vi "主界面.vi"() -> ()   [LabVIEW 2010]
uses:
  全局量/试验配置信息.vi
  全局量/全局_配置.vi
  全局量/自动测试结果.vi
panel:
  in  "进度提示":string
  in  "加载配置文件列表":u16(ring)
  out "配置文件路径":path
  out "配置文件目录":path
  in  "通道及参数配置":bool
  in  "?":enum32{"板卡类型1", "板卡类型2"}(tab)
  in  "单选_数字量输入":bool
  in  "单选_数字量输出":bool
  in  "单选_DSP输入":bool
  in  "单选_CAN检测":bool
  in  "单选_LAN检测":bool
  in  "单选_R232检测":bool
  in  "btn_数字输出":bool
  in  "btn_DSP输入":bool
  in  "btn_CAN总线":bool
  in  "btn_LAN总线":bool
  in  "btn_R232_485总线":bool
  in  "btn_开始检测":bool
  in  "btn_数字输入":bool
  in  "单选_R485检测":bool
  in  "单选_AD输入":bool
  out "数字量输入检测":bool
  out "数字量输出检测":bool
  out "模拟量DSP输入检测":bool
  out "模拟量AD输入检测":bool
  out "CAN总线检测":bool
  out "LAN总线检测":bool
  out "RS232总线检测":bool
  out "RS485总线检测":bool
  in  "btn_自动开始检测类型2":bool
  in  "函数类型 4":bool caption="y =f4(A1sin(2*π*A2)x+A3)"
  in  "函数类型 3":bool caption="y =f3(x)"
  in  "函数类型 2":bool caption="y =f2(x,A1,A2,t)"
  in  "函数类型 1":bool caption="y =f1(A1*x+A2)"
  out "函数类型4检测":bool
  out "函数类型3检测":bool
  out "函数类型2检测":bool
  out "函数类型1检测":bool
  in  "单选_函数类型4":bool
  in  "单选_函数类型3":bool
  in  "单选_函数类型2":bool
  in  "单选_函数类型1":bool
  in  "进度每次增加数":dbl
  in  "btn_二维码识别":bool
  out "退出？":bool
  in  "btn_退出":bool
  in  "btn_报告管理":bool
  in  "str_测试地点":string
  in  "str_测试人员":string
  in  "str_测试编号":string
  in  "str_报告编号":string
  # "板卡综合测试装置"
  # "板 卡 测 试 信 息"
  # "试验报告编号："
  # "测试板卡编号："
  # "板卡类型："
  # "测试人员："
  # "测试地点："
  # "自动测试"
  # "分步测试"
  # "测试\n项\n目"
  # "分步测试"
  # "自动测试"
  # "测试\n项\n目"
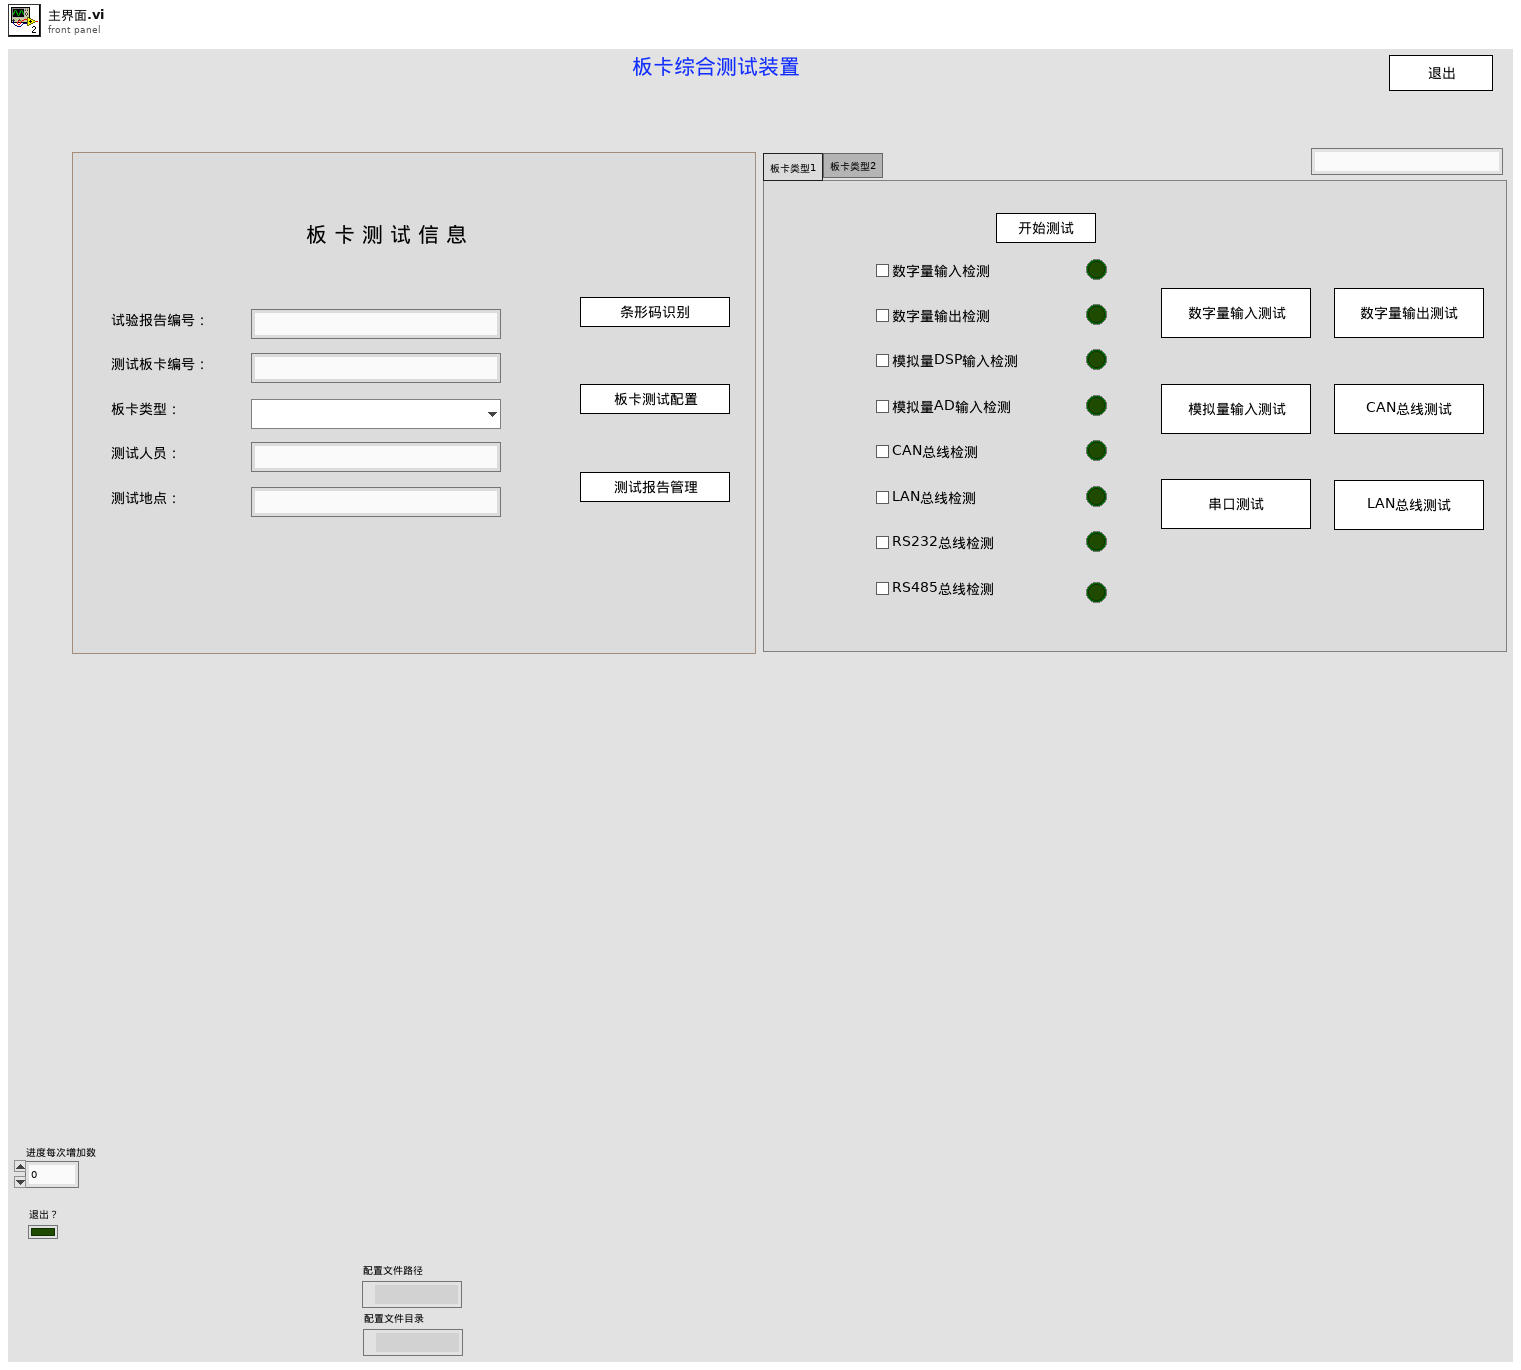
[diagram p1: front panel]
types:
  T1 = cluster{"数字量输入信号路数":i32, "数字量输出信号路数":i32, "DSP模拟量输入信号路数":u32, "DSP模拟量输入信号幅值":u32, "AD模拟量输入信号路数":u32, "AD模拟量输入信号幅值":u32, "RS232端口":u32, "RS232通信路数":u32, "RS232波特率":dbl, "RS485端口":u32, "RS485通信路数":u32, "RS485波特率":u32, "CAN通信路数":i32, "CAN波特率":u32, "以太网选择?":bool, "控制板IP":string, "以太网端口":u32}
  T2 = cluster{"str_报告编号":string, "str_测试编号":string, "RingText.Text":string, "str_测试人员":string, "str_测试地点":string}
  T3 = enum8{"Enabled", "Disabled", "Disabled and Grayed Out"}
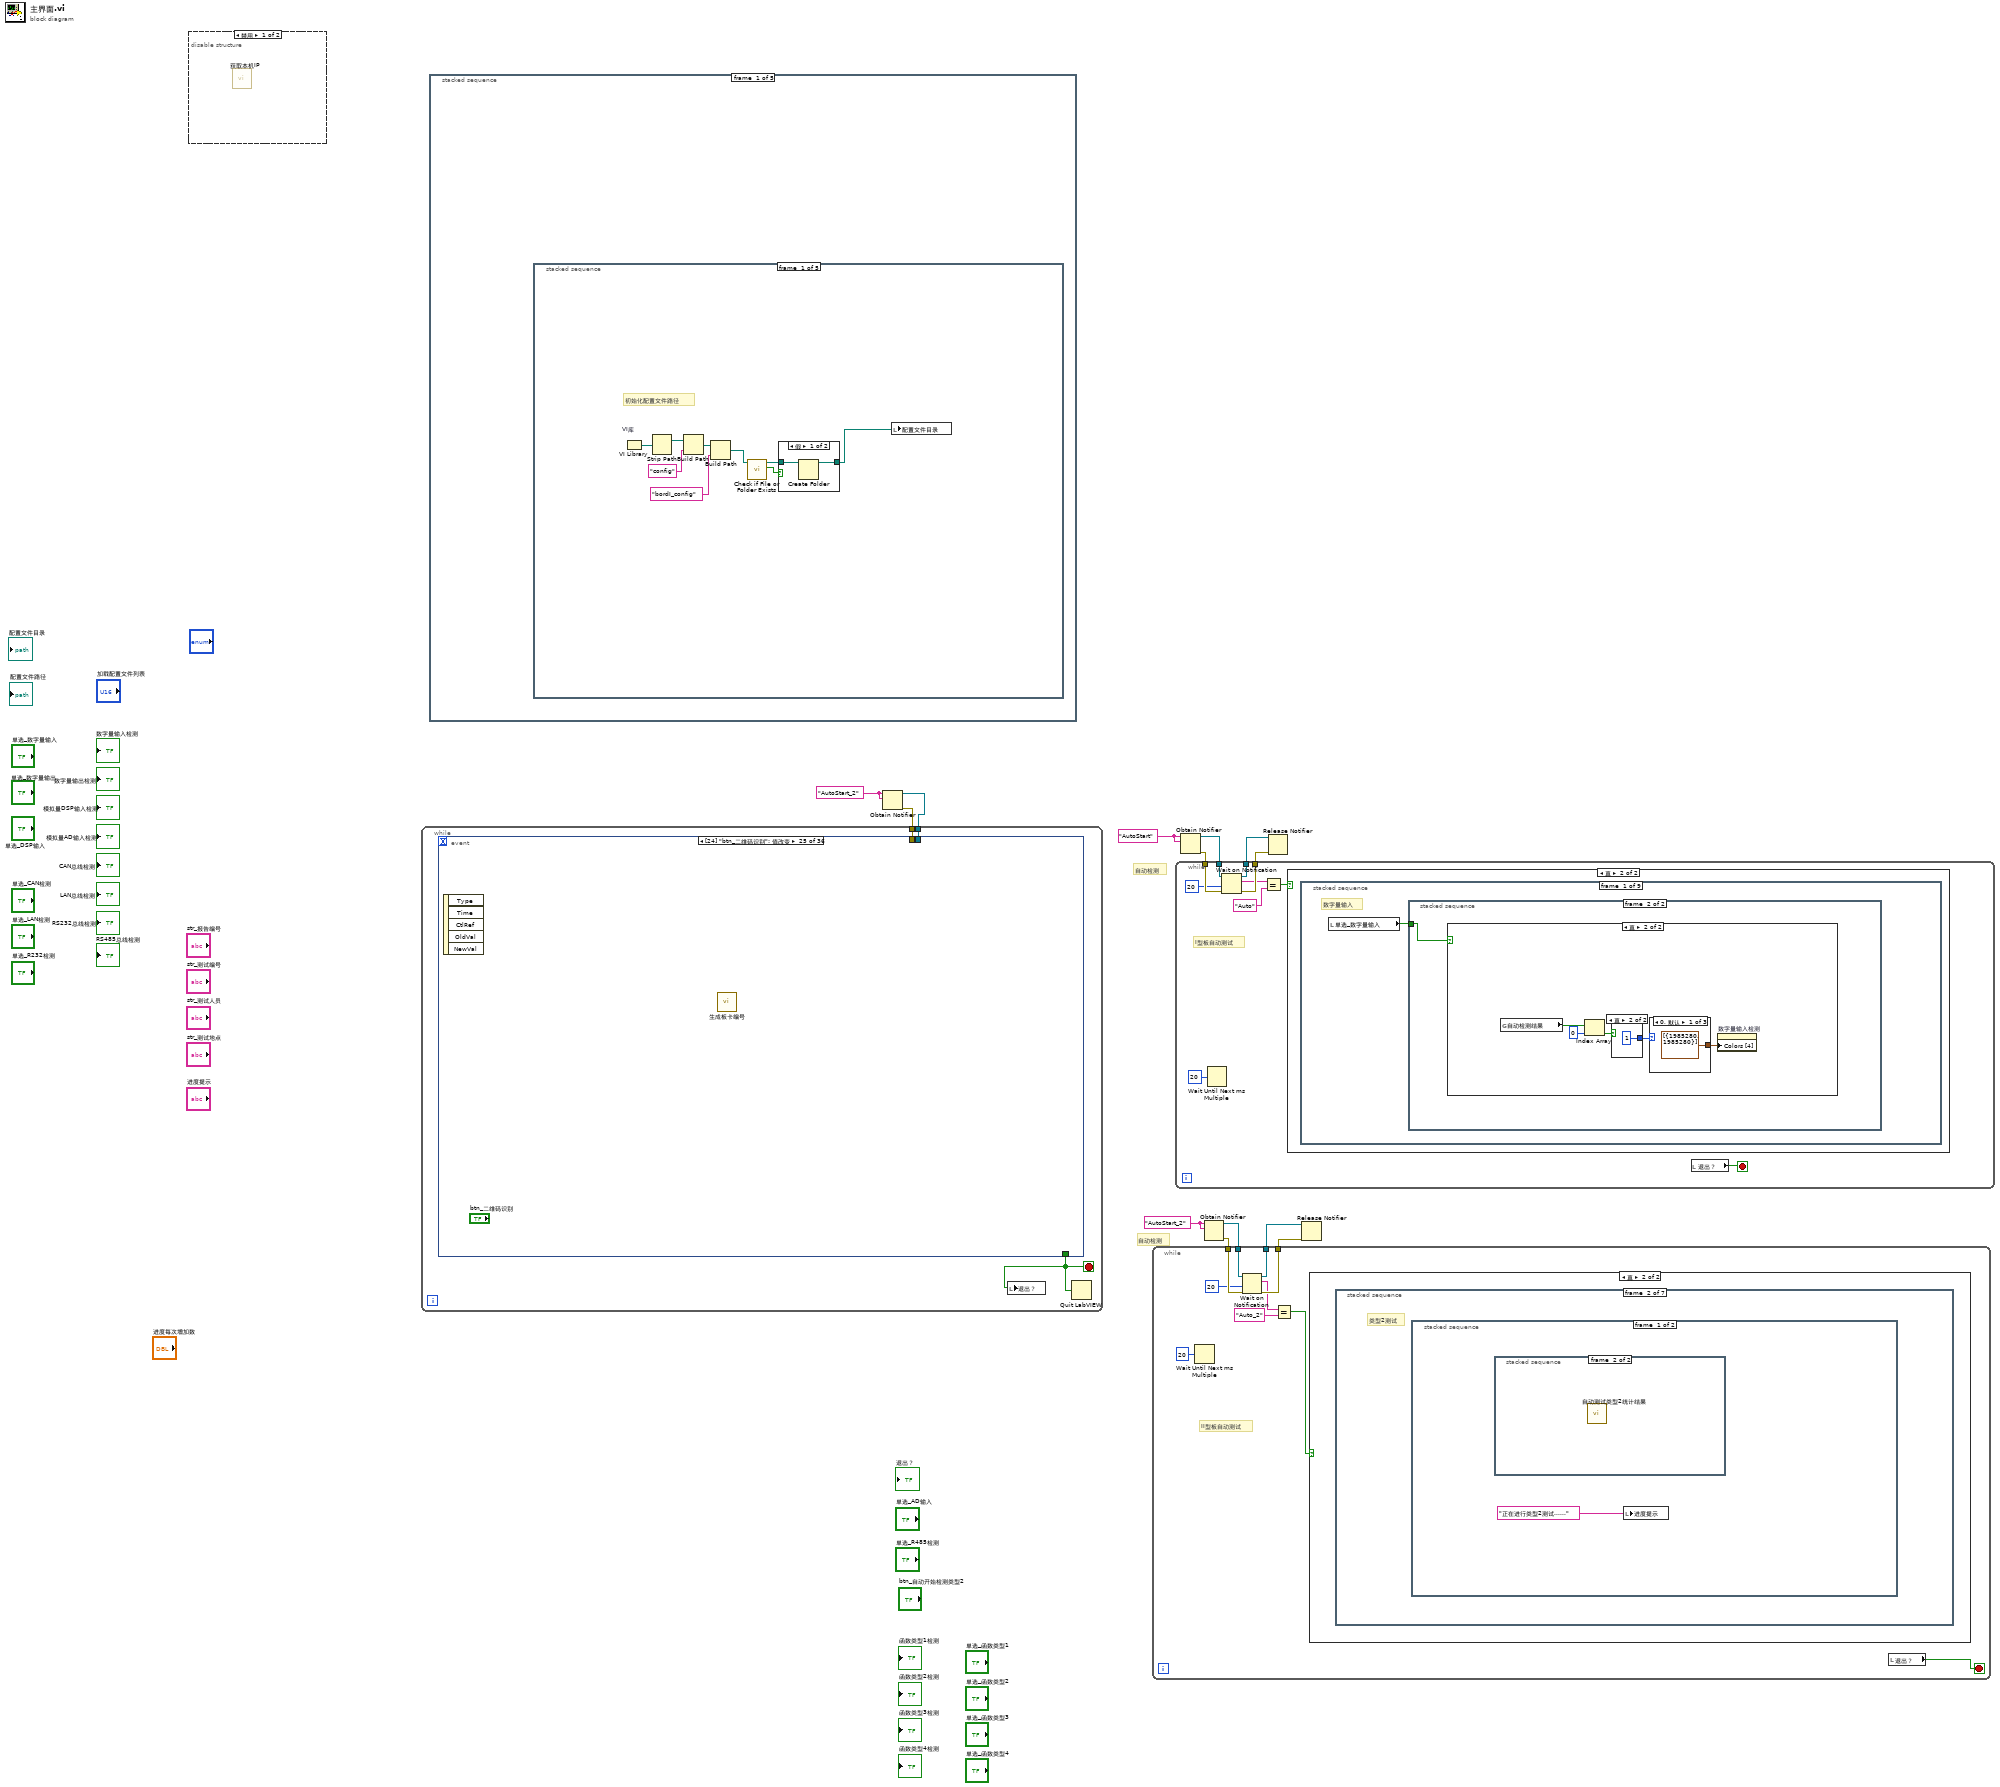
[diagram p0: block diagram]
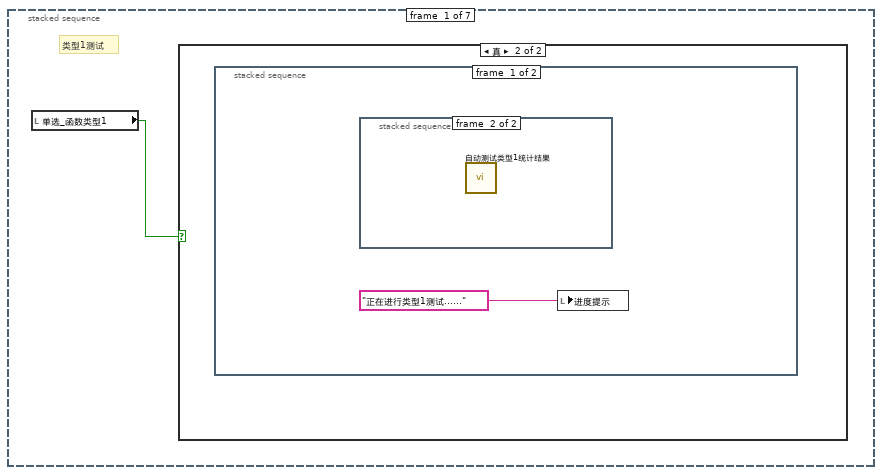
[diagram p4: hidden frame]
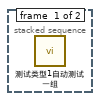
[diagram p6: hidden frame]
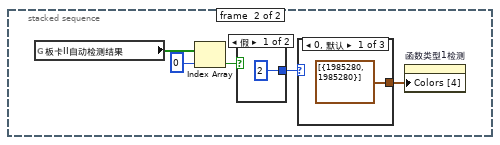
[diagram p7: hidden frame]
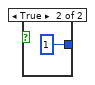
[diagram p8: hidden frame]
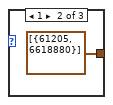
[diagram p9: hidden frame]
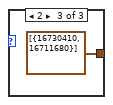
[diagram p10: hidden frame]
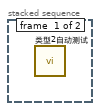
[diagram p11: hidden frame]
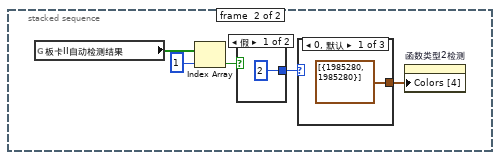
[diagram p12: hidden frame]
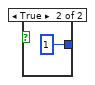
[diagram p13: hidden frame]
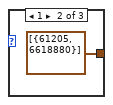
[diagram p14: hidden frame]
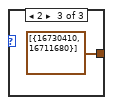
[diagram p15: hidden frame]
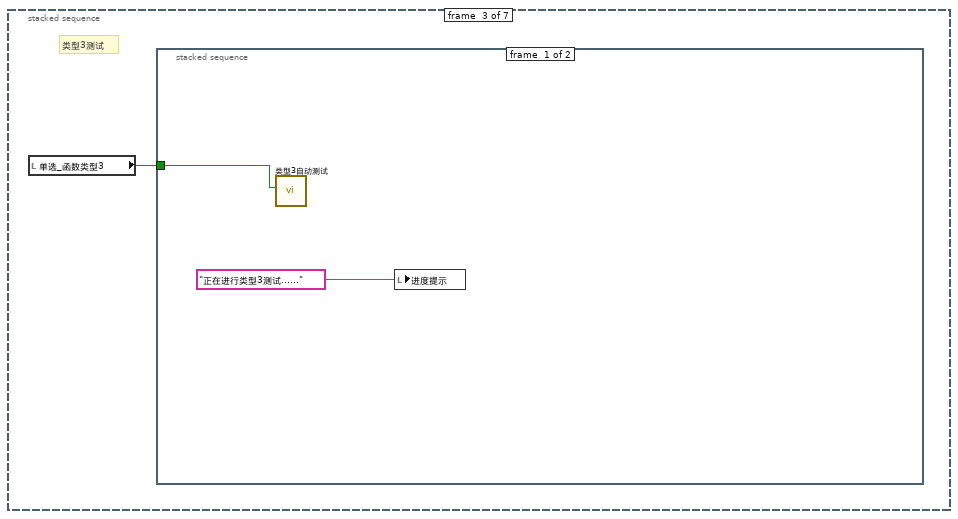
[diagram p16: hidden frame]
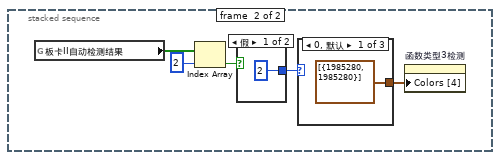
[diagram p17: hidden frame]
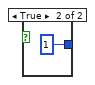
[diagram p18: hidden frame]
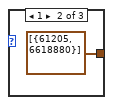
[diagram p19: hidden frame]
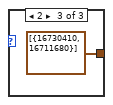
[diagram p20: hidden frame]
diagram:
  w3 = "AutoStart_2" ("名称（未命名）")
  w8 = "AutoStart_2" ("名称（未命名）")
  w13 = "AutoStart" ("名称（未命名）")
  # "自动检测"
  # "自动检测"
  n1 = disable-structure shown="禁用" {
    frame Disabled {
      n2 = call "获取本机IP.vi"() -> ()  [unwired: 9 in, 3 out]
    }
    frame Enabled {
    }
  }
  n3 = stacked-sequence {
    frame #0 {
      n4 = stacked-sequence {
        frame #0 {
          # "初始化配置文件路径"
          n5 = VI Library "VI库"() -> (path=w22:path)
          n6 = Strip Path(path=w22) -> (stripped path=w21:path)  [unwired: 1 out]
          n7 = Build Path(base path=w21, name or relative path="config" ("名称或相对路径")) -> (appended path=w19:path)
          n8 = Build Path(base path=w19, name or relative path="bordI_config" ("名称或相对路径")) -> (appended path=w15:path)
          n9 = call <vilib>:"Check if File or Folder Exists.vi"("path"=w15) -> ("file or folder exists?"=w16:bool, "dup path"=w17:path)  [unwired: 8 in, 1 out]
          n10 = case shown="假" w16 {
            tunnel: w17 -> [w23 w25]
            tunnel: [w24 w25] -> w14
            frame False {
              n11 = Create Folder(path (use dialog)=w23) -> (created path=w24:path)  [unwired: 2 in, 2 out]
            }
            frame True {
            }
          }
          n12 = local write "配置文件目录"(w14) -> ()
        }
        frame #1 {
          # "遍历配置文件目录"
          n13 = local read "配置文件目录"() -> (w27:path)
          n14 = call "罗列目录配置文件.vi"("路径"=w27) -> ("数组"=w26:string[])  [unwired: 10 in]
          n15 = property on="加载配置文件列表" class="Ring (严格)"("Strings []"=w26) -> ()  [unwired: 2 in, 2 out]
        }
        frame #2 {
          n16 = property on="加载配置文件列表" class="Ring (严格)"() -> ("RingText.Text"=w28:string)  [unwired: 2 in, 2 out]
          n17 = global write "试验配置信息.vi" "控制板类型"(w28) -> ()
        }
        frame #3 {
          # "待读取配置文件路径"
          n18 = local read "配置文件目录"() -> (w31:path)
          n19 = global read "试验配置信息.vi" "控制板类型"() -> (w29:string)
          n20 = Build Path(base path=w31, name or relative path=w29) -> (appended path=w30:path)
          n21 = local write "配置文件路径"(w30) -> ()
        }
        frame #4 {
          n22 = disable-structure shown="禁用" {
            frame Disabled {
              n23 = local read "配置文件路径"() -> (w40:path)
              n24 = call "函数测试配置文件读取.vi"("配置文件路径"=w40) -> ("类型1路数"=w35:i32, "类型2路数"=w34:i32, "类型3路数"=w33:i32, "类型4路数"=w32:i32, "D_IN_1"=w39:string[][], "D_IN_2"=w38:string[][], "D_IN_3"=w37:string[][], "D_IN_4"=w36:string[][])  [unwired: 11 in]
              n25 = global write "试验配置信息.vi" "自测类型4路数"(w32) -> ()
              n26 = global write "试验配置信息.vi" "D_IN_1"(w39) -> ()
              n27 = global write "试验配置信息.vi" "D_IN_2"(w38) -> ()
              n28 = global write "试验配置信息.vi" "D_IN_3"(w37) -> ()
              n29 = global write "试验配置信息.vi" "D_IN_4"(w36) -> ()
              n30 = global write "试验配置信息.vi" "自测类型1路数"(w35) -> ()
              n31 = global write "试验配置信息.vi" "自测类型2路数"(w34) -> ()
              n32 = global write "试验配置信息.vi" "自测类型3路数"(w33) -> ()
            }
            frame Enabled {
            }
          }
        }
      }
    }
    frame #1 {
      n33 = global read "试验配置信息.vi" "控制板类型"() -> (w43:string)
      n34 = global write "全局_配置.vi" "CAN打开标志"(FALSE ("CAN打开标志")) -> ()
      n35 = local write "加载配置文件列表"(u16 0) -> ()
      n36 = call "读写配置文件.vi"("文件名称"=w43, "m_bRead"=TRUE) -> ("BoardConfig_output"=w56:T1)  [unwired: 9 in]
      n37 = global write "试验配置信息.vi" "配置文件序号"(u16 0 ("配置文件序号")) -> ()
      n38 = Unbundle By Name(w56) -> ("数字量输入信号路数"=w50:i32, "数字量输出信号路数"=w49:i32, "DSP模拟量输入信号路数"=w48:u32, "DSP模拟量输入信号幅值"=w54:u32, "AD模拟量输入信号路数"=w47:u32, "AD模拟量输入信号幅值"=w51:u32, "RS232通信路数"=w46:u32, "RS232波特率"=w55:dbl, "RS485通信路数"=w45:u32, "CAN通信路数"=w44:i32)  [unwired: 7 out]
      n39 = global write "全局_配置.vi" "BoardConfig"(w56) -> ()
      n40 = case shown="0, 默认" w54 {
        tunnel: [3.3 10.0 24.0] -> w53
        frame 0, Default {
        }
        frame 1 {
        }
        frame 2 {
        }
      }
      n41 = case shown="2" w51 {
        tunnel: [6.0 10.0 24.0] -> w52
        frame 0, Default {
        }
        frame 1 {
        }
        frame 2 {
        }
      }
      n42 = global write "全局_配置.vi" "模拟量误差"(w55) -> ()
      n43 = global write "全局_配置.vi" "数字量输入路数"(w50) -> ()
      n44 = global write "全局_配置.vi" "数字量输出路数"(w49) -> ()
      n45 = global write "全局_配置.vi" "dsp模拟量输入路数"(w48) -> ()
      n46 = global write "全局_配置.vi" "ad模拟量输入路数"(w47) -> ()
      n47 = global write "试验配置信息.vi" "自测CAN路数"(w44) -> ()
      n48 = global write "全局_配置.vi" "R485路数"(w45) -> ()
      n49 = global write "全局_配置.vi" "CAN波特率"(u16 250 ("CAN波特率")) -> ()
      n50 = global write "全局_配置.vi" "R232路数"(w46) -> ()
      n51 = global write "全局_配置.vi" "DSP模拟量量程范围"(w53) -> ()
      n52 = global write "全局_配置.vi" "ARM模拟量量程范围"(w52) -> ()
      n53 = disable-structure shown="禁用" {
        frame Disabled {
          (unwired) "192.168.1.15" ("本机IP")
          (unwired) "192.168.1.10" ("控制板IP")
        }
        frame Enabled {
        }
      }
      n54 = global write "全局_配置.vi" "CAN发送帧数"(u32 100 ("CAN发送帧数")) -> ()
      n55 = global write "全局_配置.vi" "超时时间_10"(10.0 ("超时时间_102")) -> ()
      n56 = global write "全局_配置.vi" "超时时间_10"(5.0 ("超时时间_10")) -> ()
      n57 = global write "全局_配置.vi" "超时时间_2"(2.0 ("超时时间_2")) -> ()
      n58 = global write "全局_配置.vi" "控制板端口"(u16 6600 ("控制板端口")) -> ()
      n59 = global write "全局_配置.vi" "本机端口"(u16 6601 ("本机端口")) -> ()
      n60 = global write "全局_配置.vi" "本机IP"("192.168.1.15" ("本机IP")) -> ()
      n61 = global write "全局_配置.vi" "控制板IP"("192.168.1.10" ("控制板IP")) -> ()
    }
    frame #2 {
      n62 = global write "试验配置信息.vi" "自测485路数"(1 ("自测485路数")) -> ()
      n63 = global write "试验配置信息.vi" "自测LAN路数"(1 ("自测LAN路数")) -> ()
    }
    frame #3 {
      w105 = TRUE ("单选_数字量输入")
      # "自动测试"
      n64 = case shown="0, 默认" 0 {
        tunnel: [cluster{u32, u32}[] [{1985280, 1985280}] cluster{u32, u32}[] [{61205, 6618880}] cluster{u32, u32}[] [{16730410, 16711680}]] -> w104
        frame 0, Default {
        }
        frame 1 {
        }
        frame 2 {
        }
      }
      n65 = property on="数字量输入检测" class="Bool (严格)"("Colors [4]"=w104) -> ()  [unwired: 2 in, 2 out]
      n66 = property on="数字量输出检测" class="Bool (严格)"("Colors [4]"=w104) -> ()  [unwired: 2 in, 2 out]
      n67 = property on="模拟量AD输入检测" class="Bool (严格)"("Colors [4]"=w104) -> ()  [unwired: 2 in, 2 out]
      n68 = property on="CAN总线检测" class="Bool (严格)"("Colors [4]"=w104) -> ()  [unwired: 2 in, 2 out]
      n69 = global write "自动测试结果.vi" "DI自动测试结果"(string[][] [["序号", "检测内容", "结果"]] ("自动测试结果")) -> ()
      n70 = property on="LAN总线检测" class="Bool (严格)"("Colors [4]"=w104) -> ()  [unwired: 2 in, 2 out]
      n71 = property on="RS232总线检测" class="Bool (严格)"("Colors [4]"=w104) -> ()  [unwired: 2 in, 2 out]
      n72 = property on="RS485总线检测" class="Bool (严格)"("Colors [4]"=w104) -> ()  [unwired: 2 in, 2 out]
      n73 = property on="模拟量DSP输入检测" class="Bool (严格)"("Colors [4]"=w104) -> ()  [unwired: 2 in, 2 out]
      n74 = property on="函数类型1检测" class="Bool (严格)"("Colors [4]"=w104) -> ()  [unwired: 2 in, 2 out]
      n75 = property on="函数类型2检测" class="Bool (严格)"("Colors [4]"=w104) -> ()  [unwired: 2 in, 2 out]
      n76 = property on="函数类型3检测" class="Bool (严格)"("Colors [4]"=w104) -> ()  [unwired: 2 in, 2 out]
      n77 = property on="函数类型4检测" class="Bool (严格)"("Colors [4]"=w104) -> ()  [unwired: 2 in, 2 out]
      n78 = global write "试验配置信息.vi" "自测类数"(0 ("自动测试个数")) -> ()
      n79 = local write "str_报告编号"("B001001000001" ("通知")) -> ()
      n80 = local write "str_测试地点"("1号实验室" ("str_测试地点")) -> ()
      n81 = global read "试验配置信息.vi" "自测类型1路数"() -> (w91:i32)
      n82 = global read "试验配置信息.vi" "自测类型1路数"() -> (w102:i32)
      n83 = global read "试验配置信息.vi" "自测类型2路数"() -> (w99:i32)
      n84 = global read "试验配置信息.vi" "自测类型3路数"() -> (w96:i32)
      n85 = global read "试验配置信息.vi" "自测类型4路数"() -> (w93:i32)
      n86 = Initialize Array(TRUE, 5 ("维数大小"), 16 ("维数大小")) -> (w81:bool[][])
      n87 = Initialize Array(TRUE, 5 ("维数大小"), 16 ("维数大小")) -> (w86:bool[][])
      n88 = Initialize Array(0.0, w91) -> (w90:dbl[])
      n89 = Initialize Array(TRUE ("元素"), w102) -> (w103:bool[])
      n90 = Initialize Array(TRUE ("元素"), w99) -> (w98:bool[])
      n91 = Initialize Array(TRUE ("元素"), w96) -> (w97:bool[])
      n92 = Initialize Array(TRUE ("元素"), w93) -> (w92:bool[])
      n93 = Initialize Array(TRUE ("元素"), 4 ("维数大小")) -> (w111:bool[])
      n94 = Initialize Array(TRUE ("元素"), 1 ("维数大小")) -> (w110:bool[])
      n95 = local write "单选_数字量输入"(w105) -> ()
      n96 = local write "单选_数字量输出"(w105) -> ()
      n97 = local write "单选_DSP输入"(w105) -> ()
      n98 = local write "单选_CAN检测"(w105) -> ()
      n99 = local write "单选_LAN检测"(w105) -> ()
      n100 = local write "单选_R232检测"(w105) -> ()
      n101 = local write "单选_R485检测"(w105) -> ()
      n102 = local write "单选_AD输入"(w105) -> ()
      n103 = Initialize Array(TRUE ("元素"), 16 ("维数大小")) -> (w118:bool[])
      n104 = Initialize Array(TRUE ("元素"), 2 ("维数大小")) -> (w107:bool[])
      n105 = Initialize Array(TRUE ("元素"), 16 ("维数大小")) -> (w113:bool[])
      n106 = global write "自动测试结果.vi" "Auto_DO_R"(w81) -> ()
      n107 = global write "自动测试结果.vi" "Auto_DI_R"(w86) -> ()
      n108 = global write "自动测试结果.vi" "Auto_func_1_max_WC"(w90) -> ()
      n109 = global write "自动测试结果.vi" "Auto_func_1_R"(w103) -> ()
      n110 = global write "自动测试结果.vi" "Auto_func_2_R"(w98) -> ()
      n111 = global write "自动测试结果.vi" "Auto_func_3_R"(w97) -> ()
      n112 = global write "自动测试结果.vi" "Auto_func_4_R"(w92) -> ()
      n113 = global write "自动测试结果.vi" "Auto_RS485_R"(w110) -> ()
      n114 = global write "自动测试结果.vi" "Auto_RS232_R"(w107) -> ()
      n115 = global write "自动测试结果.vi" "Auto_CAN_R"(w111) -> ()
      n116 = global write "自动测试结果.vi" "Auto_DSP_R"(w118) -> ()
      n117 = global write "自动测试结果.vi" "Auto_AD_R"(w113) -> ()
      n118 = local write "单选_函数类型1"(w105) -> ()
      n119 = local write "单选_函数类型2"(w105) -> ()
      n120 = local write "单选_函数类型3"(w105) -> ()
      n121 = local write "单选_函数类型4"(w105) -> ()
    }
    frame #4 {
      n122 = call "实验配置信息读取和写入.vi"("读取写入"=FALSE) -> ("输出簇"=w140:T2)  [unwired: 8 in]
      n123 = Unbundle By Name(w140) -> ("str_报告编号"=w138:string, "str_测试编号"=w137:string, "str_测试人员"=w135:string, "str_测试地点"=w136:string)
      n124 = Initialize Array(TRUE, 8 ("维数大小")) -> (w133:bool[])
      n125 = Initialize Array(TRUE, 4 ("维数大小")) -> (w130:bool[])
      n126 = call <vilib>:"RGB to Color.vi"("B"=255 ("维数大小"), "G"=0 ("维数大小"), "R"=0 ("维数大小")) -> ("Color"=w127:u32)
      n127 = global write "试验配置信息.vi" "板卡II自动检测结果"(w130) -> ()
      n128 = local write "str_报告编号"(w138) -> ()
      n129 = local write "str_测试编号"(w137) -> ()
      n130 = property on="进度提示" class="Str"("Text.TextColor"=w127) -> ()  [unwired: 2 in, 2 out]
      n131 = local write "进度提示"("测试准备就绪......") -> ()
      n132 = global write "试验配置信息.vi" "自动检测结果"(w133) -> ()
      n133 = local write "str_测试地点"(w136) -> ()
      n134 = local write "str_测试人员"(w135) -> ()
    }
  }
  n135 = Obtain Notifier(name (unnamed)=w3, notification data type=w3) -> (notifier out=w2:refnum<notifier>, error out=w1:errorcluster)  [unwired: 2 in, 1 out]
  n136 = while {
    tunnel: w2 -> [w142]
    tunnel: w1 -> [w141]
    stop <- w143 stop-if-true
    n137 = event shown="[24] \"btn_二维码识别\": 值改变" {
      selector: _ -> [_ _ _ _ _ _ _ _ _ _ _ _ _ _ _ _ _ _ _ _ _ _ _ _ _ _ _ _ _ _ _ _ _ _ _ _]
      dyn-events: _ -> [_ _ _ _ _ _ _ _ _ _ _ _ _ _ _ _ _ _ _ _ _ _ _ _ _ _ _ _ _ _ _ _ _ _ _ _]
      timeout: _ -> [_ _ _ _ _ _ _ _ _ _ _ _ _ _ _ _ _ _ _ _ _ _ _ _ _ _ _ _ _ _ _ _ _ _ _ _]
      tunnel: [_ w144 _ _ _ _ _ _ _ _ _ _ _ _ _ _ _ _ _ _ _ _ _ _ _ _ _ _ _ _ _ _ _ _ _ _] -> w143
      tunnel: w142 -> [_ _ _ _ _ _ _ _ _ _ _ _ _ _ _ _ _ w318 _ _ _ _ _ _ _ _ _ _ _ _ _ _ _ _ _ _]
      tunnel: w141 -> [_ _ _ _ _ _ _ _ _ _ _ _ _ _ _ _ _ w317 _ _ _ _ _ _ _ _ _ _ _ _ _ _ _ _ _ _]
      event Timeout {
        n138 = event-data() -> ()  [unwired: 1 in, 2 out]
      }
      event "btn_退出": Value Change {
        n139 = event-data() -> ()  [unwired: 1 in, 5 out]
        n140 = case shown="真" "btn_退出" {
          tunnel: [FALSE TRUE] -> w144
          frame False {
          }
          frame True {
          }
        }
      }
      event "btn_报告管理": Value Change {
        n141 = event-data() -> ()  [unwired: 1 in, 5 out]
        n142 = call "测试报告管理.vi"() -> ()  [unwired: 12 in]
      }
      event "单选_数字量输入": Value Change {
        n143 = event-data() -> ("NewVal"=w148:bool)  [unwired: 1 in, 4 out]
        n144 = local write "单选_数字量输入"(w148) -> ()
      }
      event "单选_数字量输出": Value Change {
        n145 = event-data() -> ("NewVal"=w149:bool)  [unwired: 1 in, 4 out]
        n146 = local write "单选_数字量输出"(w149) -> ()
      }
      event "单选_DSP输入": Value Change {
        n147 = event-data() -> ("NewVal"=w150:bool)  [unwired: 1 in, 4 out]
        n148 = local write "单选_DSP输入"(w150) -> ()
      }
      event "单选_CAN检测": Value Change {
        n149 = event-data() -> ("NewVal"=w151:bool)  [unwired: 1 in, 4 out]
        n150 = local write "单选_CAN检测"(w151) -> ()
      }
      event "单选_LAN检测": Value Change {
        n151 = event-data() -> ("NewVal"=w152:bool)  [unwired: 1 in, 4 out]
        n152 = local write "单选_LAN检测"(w152) -> ()
      }
      event "单选_R232检测": Value Change {
        n153 = event-data() -> ("NewVal"=w153:bool)  [unwired: 1 in, 4 out]
        n154 = local write "单选_R232检测"(w153) -> ()
      }
      event "btn_数字输入": Value Change {
        n155 = event-data() -> ()  [unwired: 1 in, 5 out]
        n156 = call "数字量输入配置.vi"() -> ()  [unwired: 12 in]
      }
      event "btn_数字输出": Value Change {
        n157 = event-data() -> ()  [unwired: 1 in, 5 out]
        n158 = call "数字量输出配置.vi"() -> ()  [unwired: 12 in]
      }
      event "btn_DSP输入": Value Change {
        n159 = event-data() -> ()  [unwired: 1 in, 5 out]
        n160 = call "32路模拟量输入.vi"() -> ()  [unwired: 12 in]
      }
      event "btn_CAN总线": Value Change {
        n161 = event-data() -> ()  [unwired: 1 in, 5 out]
        n162 = call "CAN总线测试.vi"() -> ()  [unwired: 12 in]
      }
      event "btn_LAN总线": Value Change {
        n163 = event-data() -> ()  [unwired: 1 in, 5 out]
        n164 = call "以太网测试界面.vi"() -> ()  [unwired: 12 in]
      }
      event "btn_R232_485总线": Value Change {
        n165 = event-data() -> ()  [unwired: 1 in, 5 out]
        n166 = call "RS232 485发送接收.vi"() -> ()  [unwired: 12 in]
      }
      event "btn_开始检测": Value Change {
        w155 = ""
        n167 = event-data() -> ()  [unwired: 1 in, 5 out]
        n168 = local read "单选_数字量输入"() -> (w164:bool)
        n169 = local read "单选_数字量输出"() -> (w163:bool)
        n170 = local read "单选_R232检测"() -> (w159:bool)
        n171 = local read "单选_R485检测"() -> (w160:bool)
        n172 = local read "单选_CAN检测"() -> (w157:bool)
        n173 = local read "单选_LAN检测"() -> (w158:bool)
        n174 = local read "单选_DSP输入"() -> (w162:bool)
        n175 = local read "单选_AD输入"() -> (w161:bool)
        n176 = local read "str_报告编号"() -> (w175:string)
        n177 = local read "str_测试编号"() -> (w174:string)
        n178 = local read "str_测试地点"() -> (w173:string)
        n179 = local read "str_测试人员"() -> (w172:string)
        n180 = property on="加载配置文件列表" class="Ring (严格)"() -> ("RingText.Text"=w156:string)  [unwired: 2 in, 2 out]
        n181 = Not Equal?(x=w175, y=w155) -> (x != y?=w171:bool)
        n182 = Not Equal?(x=w174, y=w155) -> (x != y?=w170:bool)
        n183 = Not Equal?(x=w173, y=w155) -> (x != y?=w169:bool)
        n184 = Not Equal?(x=w172, y=w155) -> (x != y?=w168:bool)
        n185 = Not Equal?(x=w156, y=w155) -> (x != y?=w154:bool)
        n186 = global write "试验配置信息.vi" "数字量输出选择？"(w163) -> ()
        n187 = global write "试验配置信息.vi" "数字量输入选择？"(w164) -> ()
        n188 = Compound Arithmetic op=AND(w154, w171, w170, w169, w168) -> (w166:bool)
        n189 = global write "试验配置信息.vi" "DSP输入选择？"(w162) -> ()
        n190 = global write "试验配置信息.vi" "CAN选择？"(w157) -> ()
        n191 = global write "试验配置信息.vi" "LAN选择？"(w158) -> ()
        n192 = global write "试验配置信息.vi" "RS232选择？"(w159) -> ()
        n193 = global write "试验配置信息.vi" "RS485选择？"(w160) -> ()
        n194 = global write "试验配置信息.vi" "AD输入选择？"(w161) -> ()
        n195 = Compound Arithmetic op=OR(w164, w163, w162, w157, w158, w159, w160, w161) -> (w165:bool)
        n196 = And(x=w166, y=w165) -> (x .and. y?=w167:bool)
        n197 = case shown="真" w167 {
          tunnel: w166 -> [w177 _]
          tunnel: w165 -> [w176 _]
          frame False {
            n198 = case shown="假" w176 {
              frame False {
                n199 = call "显示对话框信息2"() -> ()  [unwired: 10 in, 2 out]
              }
              frame True {
              }
            }
            n200 = case shown="假" w177 {
              frame False {
                n201 = call "显示对话框信息"() -> ()  [unwired: 10 in, 2 out]
              }
              frame True {
              }
            }
          }
          frame True {
            n202 = stacked-sequence {
              frame #0 {
                n203 = property on="加载配置文件列表" class="Ring (严格)"() -> ("RingText.Text"=w179:string)  [unwired: 2 in, 2 out]
                n204 = local read "str_报告编号"() -> (w185:string)
                n205 = local read "str_测试编号"() -> (w186:string)
                n206 = local read "str_测试地点"() -> (w188:string)
                n207 = local read "str_测试人员"() -> (w187:string)
                n208 = local read "str_测试地点"() -> (w178:string)
                n209 = local read "str_报告编号"() -> (w183:string)
                n210 = local read "str_测试编号"() -> (w182:string)
                n211 = local read "str_测试人员"() -> (w180:string)
                n212 = global write "试验配置信息.vi" "报告编号"(w185) -> ()
                n213 = global write "试验配置信息.vi" "控制板编号"(w186) -> ()
                n214 = global write "试验配置信息.vi" "测试地点"(w188) -> ()
                n215 = global write "试验配置信息.vi" "测试人员"(w187) -> ()
                n216 = Bundle("str_报告编号"=w183, "str_测试编号"=w182, "RingText.Text"=w179, "str_测试人员"=w180, "str_测试地点"=w178) -> (w181:T2)  [unwired: 1 in]
                n217 = global write "试验配置信息.vi" "控制板类型"(w179) -> ()
                n218 = call "实验配置信息读取和写入.vi"("读取写入"=TRUE, "输入簇"=w181) -> ()  [unwired: 7 in, 1 out]
              }
              frame #1 {
                n219 = local read "单选_数字量输入"() -> (w197:bool)
                n220 = local read "单选_数字量输出"() -> (w196:bool)
                n221 = local read "单选_R232检测"() -> (w191:bool)
                n222 = local read "单选_R485检测"() -> (w190:bool)
                n223 = local read "单选_CAN检测"() -> (w193:bool)
                n224 = local read "单选_LAN检测"() -> (w192:bool)
                n225 = local read "单选_DSP输入"() -> (w195:bool)
                n226 = local read "单选_AD输入"() -> (w189:bool)
                n227 = Build Array(w197, w196, w195, w193, w192, w191, w190, w189) -> (w194:bool[])
                n228 = for {
                  tunnel: w194 -> [w198] mode=indexing
                  n229 = case shown="真" w198 {
                    frame False {
                    }
                    frame True {
                      n230 = global read "试验配置信息.vi" "自测类数"() -> (w200:i32)
                      n231 = Increment(x=w200) -> (x+1=w199:i32)
                      n232 = global write "试验配置信息.vi" "自测类数"(w199) -> ()
                    }
                  }
                }
              }
              frame #2 {
                n233 = global read "试验配置信息.vi" "数字量输出选择？"() -> (w207:bool)
                n234 = global read "试验配置信息.vi" "数字量输入选择？"() -> (w208:bool)
                n235 = global read "试验配置信息.vi" "AD输入选择？"() -> (w205:bool)
                n236 = global read "试验配置信息.vi" "DSP输入选择？"() -> (w206:bool)
                n237 = global read "试验配置信息.vi" "CAN选择？"() -> (w204:bool)
                n238 = global read "试验配置信息.vi" "RS232选择？"() -> (w202:bool)
                n239 = global read "试验配置信息.vi" "RS485选择？"() -> (w201:bool)
                n240 = global read "试验配置信息.vi" "LAN选择？"() -> (w203:bool)
                n241 = case shown="真" w206 {
                  tunnel: [0 w227] -> w214
                  frame False {
                  }
                  frame True {
                    n242 = global read "全局_配置.vi" "dsp模拟量输入路数"() -> (w227:u32)
                  }
                }
                n243 = case shown="真" w205 {
                  tunnel: [0 w229] -> w215
                  frame False {
                  }
                  frame True {
                    n244 = global read "全局_配置.vi" "ad模拟量输入路数"() -> (w229:u32)
                  }
                }
                n245 = case shown="真" w207 {
                  tunnel: [0 w231] -> w216
                  frame False {
                  }
                  frame True {
                    n246 = global read "全局_配置.vi" "数字量输出路数"() -> (w231:i32)
                  }
                }
                n247 = case shown="真" w208 {
                  tunnel: [0 w233] -> w217
                  frame False {
                  }
                  frame True {
                    n248 = global read "全局_配置.vi" "数字量输入路数"() -> (w233:i32)
                  }
                }
                n249 = case shown="真" w204 {
                  tunnel: [0 w225] -> w213
                  frame False {
                  }
                  frame True {
                    n250 = global read "试验配置信息.vi" "自测CAN路数"() -> (w225:i32)
                  }
                }
                n251 = case shown="真" w202 {
                  tunnel: [0 w223] -> w212
                  frame False {
                  }
                  frame True {
                    n252 = global read "全局_配置.vi" "R232路数"() -> (w223:u32)
                  }
                }
                n253 = case shown="真" w201 {
                  tunnel: [0 w221] -> w211
                  frame False {
                  }
                  frame True {
                    n254 = global read "试验配置信息.vi" "自测485路数"() -> (w221:i32)
                  }
                }
                n255 = case shown="真" w203 {
                  tunnel: [0 w219] -> w210
                  frame False {
                  }
                  frame True {
                    n256 = global read "试验配置信息.vi" "自测LAN路数"() -> (w219:i32)
                  }
                }
                n257 = Compound Arithmetic op=ADD(w217, w216, w215, w214, w213, w212, w211, w210) -> (w209:u32)
                n258 = global write "试验配置信息.vi" "自测项数"(w209) -> ()
              }
              frame #3 {
                w241 = string[][] [["序号", "检测内容", "测试结果"]] ("自动测试结果")
                n259 = global read "全局_配置.vi" "dsp模拟量输入路数"() -> (w234:u32)
                n260 = global read "全局_配置.vi" "ad模拟量输入路数"() -> (w235:u32)
                n261 = Initialize Array(0.0 ("元素"), w234) -> (w236:dbl[])
                n262 = Initialize Array(0.0 ("元素"), w235) -> (w238:dbl[])
                n263 = global write "自动测试结果.vi" "总线通信自测结果"(w241) -> ()
                n264 = global write "自动测试结果.vi" "DI自动测试结果"(w241) -> ()
                n265 = global write "自动测试结果.vi" "DO自动测试结果"(w241) -> ()
                n266 = global write "自动测试结果.vi" "Auto_DSP_max_WC"(w236) -> ()
                n267 = global write "自动测试结果.vi" "Auto_AD_max_WC"(w238) -> ()
                n268 = global write "自动测试结果.vi" "AI自动测试结果"(string[][] [["序号", "检测内容", "最大误差(%)", "测试结果"]] ("自动测试结果")) -> ()
              }
              frame #4 {
                n269 = global read "试验配置信息.vi" "自测CAN路数"() -> (w258:i32)
                n270 = global read "试验配置信息.vi" "自测485路数"() -> (w261:i32)
                n271 = Initialize Array(TRUE ("元素"), w258) -> (w259:bool[])
                n272 = Initialize Array(TRUE ("元素"), w261) -> (w260:bool[])
                n273 = Initialize Array(TRUE ("元素"), 16 ("维数大小")) -> (w254:bool[])
                n274 = Initialize Array(TRUE ("元素"), 2 ("维数大小")) -> (w264:bool[])
                n275 = Initialize Array(TRUE ("元素"), 16 ("维数大小")) -> (w256:bool[])
                n276 = Initialize Array(TRUE, 5 ("维数大小"), 16 ("维数大小")) -> (w248:bool[][])
                n277 = Initialize Array(TRUE, 5 ("维数大小"), 16 ("维数大小")) -> (w252:bool[][])
                n278 = global write "自动测试结果.vi" "Auto_RS485_R"(w260) -> ()
                n279 = global write "自动测试结果.vi" "Auto_RS232_R"(w264) -> ()
                n280 = global write "自动测试结果.vi" "Auto_CAN_R"(w259) -> ()
                n281 = global write "自动测试结果.vi" "Auto_DSP_R"(w254) -> ()
                n282 = global write "自动测试结果.vi" "Auto_AD_R"(w256) -> ()
                n283 = global write "自动测试结果.vi" "Auto_DI_R"(w248) -> ()
                n284 = global write "自动测试结果.vi" "Auto_DO_R"(w252) -> ()
              }
              frame #5 {
                w265 = ""
                n285 = global read "试验配置信息.vi" "自测类数"() -> (w272:i32)
                n286 = global read "试验配置信息.vi" "自测项数"() -> (w269:i32)
                n287 = global read "试验配置信息.vi" "自测类数"() -> (w270:i32)
                n288 = global write "自动测试结果.vi" "数字量输入概述"(w265) -> ()
                n289 = global write "自动测试结果.vi" "数字量输出概述"(w265) -> ()
                n290 = global write "自动测试结果.vi" "模拟量DSP概述"(w265) -> ()
                n291 = global write "自动测试结果.vi" "模拟量AD概述结果"(w265) -> ()
                n292 = global write "自动测试结果.vi" "串口RS232测试概述"(w265) -> ()
                n293 = global write "自动测试结果.vi" "串口RS485测试概述"(w265) -> ()
                n294 = global write "自动测试结果.vi" "CAN测试概述"(w265) -> ()
                n295 = global write "自动测试结果.vi" "CAN测试概述"(w265) -> ()
                n296 = global write "自动测试结果.vi" "以太网测试概述"(w265) -> ()
                n297 = Divide(x=100, y=w272) -> (x/y=w274:dbl)
                n298 = property on="进度每次增加数" class="DigNum (严格)"("Value"=w274) -> ()  [unwired: 2 in, 2 out]
                n299 = Format Into String(format string="本报告测试项目共%d类，测试项总计%d项，其中：" ("时间格式字符串(%c)"), w270, w269) -> (resulting string=w267:string)  [unwired: 2 in, 1 out]
                n300 = Concatenate Strings(w267, "\r") -> (w268:string)
                n301 = global write "自动测试结果.vi" "自测总概述"(w268) -> ()
              }
              frame #6 {
                w277 = "AutoStart" ("名称（未命名）")
                n302 = Obtain Notifier(name (unnamed)=w277, notification data type=w277) -> (notifier out=w276:refnum<notifier>)  [unwired: 2 in, 2 out]
                n303 = local write "进度提示"("正在测试中，请耐心等待结果......") -> ()
                n304 = Send Notification(notification="Auto" ("通知"), notifier=w276) -> ()  [unwired: 1 in, 2 out]
              }
              frame #7 {
                w279 = T3."Disabled and Grayed Out" ("禁用")
                n305 = property on="btn_数字输入" class="Bool"("DisabledEnum"=w279) -> ()  [unwired: 2 in, 2 out]
                n306 = property on="btn_数字输出" class="Bool"("DisabledEnum"=w279) -> ()  [unwired: 2 in, 2 out]
                n307 = property on="btn_DSP输入" class="Bool"("DisabledEnum"=w279) -> ()  [unwired: 2 in, 2 out]
                n308 = property on="btn_CAN总线" class="Bool"("DisabledEnum"=w279) -> ()  [unwired: 2 in, 2 out]
                n309 = property on="btn_R232_485总线" class="Bool"("DisabledEnum"=w279) -> ()  [unwired: 2 in, 2 out]
                n310 = property on="btn_LAN总线" class="Bool"("DisabledEnum"=w279) -> ()  [unwired: 2 in, 2 out]
                n311 = property on="函数类型 1" class="Bool"("DisabledEnum"=w279) -> ()  [unwired: 2 in, 2 out]
                n312 = property on="函数类型 2" class="Bool"("DisabledEnum"=w279) -> ()  [unwired: 2 in, 2 out]
                n313 = property on="函数类型 3" class="Bool"("DisabledEnum"=w279) -> ()  [unwired: 2 in, 2 out]
                n314 = property on="函数类型 4" class="Bool"("DisabledEnum"=w279) -> ()  [unwired: 2 in, 2 out]
                n315 = property on="btn_自动开始检测类型2" class="Bool"("DisabledEnum"=w279) -> ()  [unwired: 2 in, 2 out]
              }
            }
          }
        }
      }
      event "加载配置文件列表": Value Change {
        n316 = event-data() -> ()  [unwired: 1 in, 5 out]
        n317 = stacked-sequence {
          frame #0 {
            n318 = property on="加载配置文件列表" class="Ring (严格)"() -> ("RingText.Text"=w280:string)  [unwired: 2 in, 2 out]
            n319 = global write "试验配置信息.vi" "控制板类型"(w280) -> ()
          }
          frame #1 {
            # "待读取配置文件路径"
            n320 = local read "配置文件目录"() -> (w281:path)
            n321 = global read "试验配置信息.vi" "控制板类型"() -> (w283:string)
            n322 = Build Path(base path=w281, name or relative path=w283) -> (appended path=w282:path)
            n323 = local write "配置文件路径"(w282) -> ()
          }
          frame #2 {
            n324 = local read "配置文件路径"() -> (w288:path)
            n325 = call "函数测试配置文件读取.vi"("配置文件路径"=w288) -> ("类型1路数"=w287:i32, "类型2路数"=w286:i32, "类型3路数"=w285:i32, "类型4路数"=w284:i32, "D_IN_1"=w289:string[][], "D_IN_2"=w290:string[][], "D_IN_3"=w291:string[][], "D_IN_4"=w292:string[][])  [unwired: 11 in]
            n326 = global write "试验配置信息.vi" "自测类型4路数"(w284) -> ()
            n327 = global write "试验配置信息.vi" "D_IN_1"(w289) -> ()
            n328 = global write "试验配置信息.vi" "D_IN_2"(w290) -> ()
            n329 = global write "试验配置信息.vi" "D_IN_3"(w291) -> ()
            n330 = global write "试验配置信息.vi" "D_IN_4"(w292) -> ()
            n331 = global write "试验配置信息.vi" "自测类型1路数"(w287) -> ()
            n332 = global write "试验配置信息.vi" "自测类型2路数"(w286) -> ()
            n333 = global write "试验配置信息.vi" "自测类型3路数"(w285) -> ()
          }
          frame #3 {
            n334 = global read "试验配置信息.vi" "控制板类型"() -> (w301:string)
            n335 = call "读写配置文件.vi"("文件名称"=w301, "m_bRead"=TRUE) -> ("BoardConfig_output"=w302:T1)  [unwired: 9 in]
            n336 = global write "全局_配置.vi" "BoardConfig"(w302) -> ()
            n337 = Unbundle By Name(w302) -> ("数字量输入信号路数"=w299:i32, "数字量输出信号路数"=w298:i32, "DSP模拟量输入信号路数"=w297:u32, "DSP模拟量输入信号幅值"=w304:u32, "AD模拟量输入信号路数"=w296:u32, "AD模拟量输入信号幅值"=w307:u32, "RS232通信路数"=w295:u32, "RS232波特率"=w303:dbl, "RS485通信路数"=w294:u32, "CAN通信路数"=w293:i32)  [unwired: 7 out]
            n338 = case shown="0, 默认" w304 {
              tunnel: [3.3 10.0 24.0] -> w305
              frame 0, Default {
              }
              frame 1 {
              }
              frame 2 {
              }
            }
            n339 = case shown="2" w307 {
              tunnel: [6.0 10.0 24.0] -> w306
              frame 0, Default {
              }
              frame 1 {
              }
              frame 2 {
              }
            }
            n340 = global write "全局_配置.vi" "模拟量误差"(w303) -> ()
            n341 = global write "全局_配置.vi" "dsp模拟量输入路数"(w297) -> ()
            n342 = global write "全局_配置.vi" "数字量输出路数"(w298) -> ()
            n343 = global write "全局_配置.vi" "数字量输入路数"(w299) -> ()
            n344 = global write "全局_配置.vi" "ad模拟量输入路数"(w296) -> ()
            n345 = global write "试验配置信息.vi" "自测CAN路数"(w293) -> ()
            n346 = global write "全局_配置.vi" "R485路数"(w294) -> ()
            n347 = global write "全局_配置.vi" "R232路数"(w295) -> ()
            n348 = global write "全局_配置.vi" "DSP模拟量量程范围"(w305) -> ()
            n349 = global write "全局_配置.vi" "ARM模拟量量程范围"(w306) -> ()
          }
        }
      }
      event "btn_自动开始检测类型2": Value Change {
        w315 = ""
        n350 = event-data() -> ()  [unwired: 1 in, 5 out]
        n351 = local read "单选_函数类型1"() -> (w325:bool)
        n352 = local read "单选_函数类型2"() -> (w324:bool)
        n353 = local read "单选_函数类型3"() -> (w323:bool)
        n354 = local read "单选_函数类型4"() -> (w322:bool)
        n355 = local read "str_报告编号"() -> (w333:string)
        n356 = local read "str_测试编号"() -> (w332:string)
        n357 = local read "str_测试地点"() -> (w331:string)
        n358 = local read "str_测试人员"() -> (w330:string)
        n359 = property on="加载配置文件列表" class="Ring (严格)"() -> ("RingText.Text"=w316:string)  [unwired: 2 in, 2 out]
        n360 = Not Equal?(x=w316, y=w315) -> (x != y?=w314:bool)
        n361 = Not Equal?(x=w333, y=w315) -> (x != y?=w329:bool)
        n362 = Not Equal?(x=w332, y=w315) -> (x != y?=w328:bool)
        n363 = Not Equal?(x=w331, y=w315) -> (x != y?=w327:bool)
        n364 = Not Equal?(x=w330, y=w315) -> (x != y?=w326:bool)
        n365 = global write "试验配置信息.vi" "测试类型1选择？"(w325) -> ()
        n366 = global write "试验配置信息.vi" "测试类型2选择？"(w324) -> ()
        n367 = global write "试验配置信息.vi" "测试类型3选择？"(w323) -> ()
        n368 = global write "试验配置信息.vi" "测试类型4选择？"(w322) -> ()
        n369 = Compound Arithmetic op=AND(w314, w329, w328, w327, w326) -> (w320:bool)
        n370 = Compound Arithmetic op=OR(w325, w324, w323, w322) -> (w319:bool)
        n371 = And(x=w320, y=w319) -> (x .and. y?=w321:bool)
        n372 = case shown="真" w321 {
          tunnel: w320 -> [w335 _]
          tunnel: w319 -> [w334 _]
          tunnel: w318 -> [_ w337]
          tunnel: w317 -> [_ w336]
          frame False {
            n373 = case shown="假" w335 {
              frame False {
                n374 = call "显示对话框信息3"() -> ()  [unwired: 10 in, 2 out]
              }
              frame True {
              }
            }
            n375 = case shown="假" w334 {
              frame False {
                n376 = call "显示对话框信息4"() -> ()  [unwired: 10 in, 2 out]
              }
              frame True {
              }
            }
          }
          frame True {
            n377 = stacked-sequence {
              tunnel: w337 -> [_ _ _ _ _ w399 _]
              tunnel: w336 -> [_ _ _ _ _ w398 _]
              frame #0 {
                n378 = property on="加载配置文件列表" class="Ring (严格)"() -> ("RingText.Text"=w341:string)  [unwired: 2 in, 2 out]
                n379 = local read "str_测试人员"() -> (w339:string)
                n380 = local read "str_报告编号"() -> (w345:string)
                n381 = local read "str_测试编号"() -> (w346:string)
                n382 = local read "str_测试地点"() -> (w348:string)
                n383 = local read "str_测试人员"() -> (w347:string)
                n384 = local read "str_测试地点"() -> (w338:string)
                n385 = local read "str_报告编号"() -> (w343:string)
                n386 = local read "str_测试编号"() -> (w342:string)
                n387 = global write "试验配置信息.vi" "报告编号"(w345) -> ()
                n388 = global write "试验配置信息.vi" "控制板编号"(w346) -> ()
                n389 = global write "试验配置信息.vi" "测试地点"(w348) -> ()
                n390 = global write "试验配置信息.vi" "测试人员"(w347) -> ()
                n391 = Bundle("str_报告编号"=w343, "str_测试编号"=w342, "RingText.Text"=w341, "str_测试人员"=w339, "str_测试地点"=w338) -> (w340:T2)  [unwired: 1 in]
                n392 = global write "试验配置信息.vi" "控制板类型"(w341) -> ()
                n393 = call "实验配置信息读取和写入.vi"("读取写入"=TRUE, "输入簇"=w340) -> ()  [unwired: 7 in, 1 out]
              }
              frame #1 {
                n394 = local read "单选_函数类型1"() -> (w353:bool)
                n395 = local read "单选_函数类型2"() -> (w352:bool)
                n396 = local read "单选_函数类型3"() -> (w351:bool)
                n397 = local read "单选_函数类型4"() -> (w350:bool)
                n398 = Build Array(w353, w352, w351, w350) -> (w349:bool[])
                n399 = for {
                  tunnel: w349 -> [w354] mode=indexing
                  n400 = case shown="真" w354 {
                    frame False {
                    }
                    frame True {
                      n401 = global read "试验配置信息.vi" "自测类数"() -> (w356:i32)
                      n402 = Increment(x=w356) -> (x+1=w355:i32)
                      n403 = global write "试验配置信息.vi" "自测类数"(w355) -> ()
                    }
                  }
                }
              }
              frame #2 {
                n404 = global read "试验配置信息.vi" "测试类型1选择？"() -> (w365:bool)
                n405 = global read "试验配置信息.vi" "测试类型2选择？"() -> (w364:bool)
                n406 = global read "试验配置信息.vi" "测试类型3选择？"() -> (w363:bool)
                n407 = global read "试验配置信息.vi" "测试类型4选择？"() -> (w362:bool)
                n408 = case shown="真" w365 {
                  tunnel: [0 w373] -> w361
                  frame False {
                  }
                  frame True {
                    n409 = global read "试验配置信息.vi" "自测类型1路数"() -> (w373:i32)
                  }
                }
                n410 = case shown="真" w363 {
                  tunnel: [0 w369] -> w359
                  frame False {
                  }
                  frame True {
                    n411 = global read "试验配置信息.vi" "自测类型3路数"() -> (w369:i32)
                  }
                }
                n412 = case shown="真" w364 {
                  tunnel: [0 w371] -> w360
                  frame False {
                  }
                  frame True {
                    n413 = global read "试验配置信息.vi" "自测类型2路数"() -> (w371:i32)
                  }
                }
                n414 = case shown="真" w362 {
                  tunnel: [0 w367] -> w358
                  frame False {
                  }
                  frame True {
                    n415 = global read "试验配置信息.vi" "自测类型4路数"() -> (w367:i32)
                  }
                }
                n416 = Compound Arithmetic op=ADD(w361, w360, w359, w358) -> (w357:i32)
                n417 = global write "试验配置信息.vi" "自测项数"(w357) -> ()
              }
              frame #3 {
                n418 = global read "试验配置信息.vi" "自测类型1路数"() -> (w378:i32)
                n419 = global read "试验配置信息.vi" "自测类型2路数"() -> (w381:i32)
                n420 = global read "试验配置信息.vi" "自测类型3路数"() -> (w384:i32)
                n421 = global read "试验配置信息.vi" "自测类型4路数"() -> (w387:i32)
                n422 = global read "试验配置信息.vi" "自测类型1路数"() -> (w374:i32)
                n423 = Initialize Array(TRUE ("元素"), w378) -> (w377:bool[])
                n424 = Initialize Array(TRUE ("元素"), w381) -> (w382:bool[])
                n425 = Initialize Array(TRUE ("元素"), w384) -> (w383:bool[])
                n426 = Initialize Array(TRUE ("元素"), w387) -> (w388:bool[])
                n427 = Initialize Array(0.0, w374) -> (w376:dbl[])
                n428 = global write "自动测试结果.vi" "Auto_func_1_R"(w377) -> ()
                n429 = global write "自动测试结果.vi" "Auto_func_2_R"(w382) -> ()
                n430 = global write "自动测试结果.vi" "Auto_func_3_R"(w383) -> ()
                n431 = global write "自动测试结果.vi" "Auto_func_4_R"(w388) -> ()
                n432 = global write "自动测试结果.vi" "Auto_func_1_max_WC"(w376) -> ()
              }
              frame #4 {
                w389 = string[][] [["序号", "输出通道", "输入通道", "测试结果", ""]] ("自动测试结果")
                w391 = ""
                n433 = global read "试验配置信息.vi" "自测项数"() -> (w395:i32)
                n434 = global read "试验配置信息.vi" "自测类数"() -> (w396:i32)
                n435 = global write "自动测试结果.vi" "测试类型1概述"(w391) -> ()
                n436 = global write "自动测试结果.vi" "测试类型2概述"(w391) -> ()
                n437 = global write "自动测试结果.vi" "测试类型3概述"(w391) -> ()
                n438 = global write "自动测试结果.vi" "测试类型4概述"(w391) -> ()
                n439 = Format Into String(format string="本报告测试项目共%d类，测试项总计%d项，其中：" ("时间格式字符串(%c)"), w396, w395) -> (resulting string=w393:string)  [unwired: 2 in, 1 out]
                n440 = global write "自动测试结果.vi" "测试类型1自动测试结果"(string[][] [["序号", "输出通道", "输入通道试结果", "最大误差(%)", "测试结果"]] ("自动测试结果")) -> ()
                n441 = global write "自动测试结果.vi" "测试类型2自动测试结果"(w389) -> ()
                n442 = global write "自动测试结果.vi" "测试类型3自动测试结果"(w389) -> ()
                n443 = global write "自动测试结果.vi" "测试类型4自动测试结果"(w389) -> ()
                n444 = Concatenate Strings(w393, "\r") -> (w394:string)
                n445 = global write "自动测试结果.vi" "自测总概述"(w394) -> ()
              }
              frame #5 {
                n446 = local write "进度提示"("正在测试中，请耐心等待结果......") -> ()
                n447 = Send Notification(notification="Auto_2" ("通知"), notifier=w399, error in (no error)=w398) -> ()  [unwired: 2 out]
              }
              frame #6 {
                w402 = T3."Disabled and Grayed Out" ("禁用")
                n448 = property on="btn_数字输入" class="Bool"("DisabledEnum"=w402) -> ()  [unwired: 2 in, 2 out]
                n449 = property on="btn_数字输出" class="Bool"("DisabledEnum"=w402) -> ()  [unwired: 2 in, 2 out]
                n450 = property on="btn_DSP输入" class="Bool"("DisabledEnum"=w402) -> ()  [unwired: 2 in, 2 out]
                n451 = property on="btn_CAN总线" class="Bool"("DisabledEnum"=w402) -> ()  [unwired: 2 in, 2 out]
                n452 = property on="btn_R232_485总线" class="Bool"("DisabledEnum"=w402) -> ()  [unwired: 2 in, 2 out]
                n453 = property on="btn_LAN总线" class="Bool"("DisabledEnum"=w402) -> ()  [unwired: 2 in, 2 out]
                n454 = property on="函数类型 1" class="Bool"("DisabledEnum"=w402) -> ()  [unwired: 2 in, 2 out]
                n455 = property on="函数类型 2" class="Bool"("DisabledEnum"=w402) -> ()  [unwired: 2 in, 2 out]
                n456 = property on="函数类型 3" class="Bool"("DisabledEnum"=w402) -> ()  [unwired: 2 in, 2 out]
                n457 = property on="函数类型 4" class="Bool"("DisabledEnum"=w402) -> ()  [unwired: 2 in, 2 out]
                n458 = property on="btn_开始检测" class="Bool"("DisabledEnum"=w402) -> ()  [unwired: 2 in, 2 out]
              }
            }
          }
        }
      }
      event "单选_函数类型1": Value Change {
        n459 = event-data() -> ("NewVal"=w403:bool)  [unwired: 1 in, 4 out]
        n460 = local write "单选_函数类型1"(w403) -> ()
      }
      event "单选_函数类型2": Value Change {
        n461 = event-data() -> ("NewVal"=w404:bool)  [unwired: 1 in, 4 out]
        n462 = local write "单选_函数类型2"(w404) -> ()
      }
      event "单选_函数类型3": Value Change {
        n463 = event-data() -> ("NewVal"=w405:bool)  [unwired: 1 in, 4 out]
        n464 = local write "单选_函数类型3"(w405) -> ()
      }
      event "单选_函数类型4": Value Change {
        n465 = event-data() -> ("NewVal"=w406:bool)  [unwired: 1 in, 4 out]
        n466 = local write "单选_函数类型4"(w406) -> ()
      }
      event "通道及参数配置": Value Change {
        n467 = event-data() -> ()  [unwired: 1 in, 5 out]
        n468 = call "通道配置模块.vi"() -> ("返回"=w407:bool)  [unwired: 11 in]
        n469 = case shown="真" w407 {
          frame False {
          }
          frame True {
            n470 = global read "试验配置信息.vi" "配置文件序号"() -> (w408:u16)
            n471 = property on="加载配置文件列表" class="Ring (严格)"("Value"=w408) -> ()  [unwired: 2 in, 2 out]
          }
        }
      }
      event "函数类型 1": Value Change {
        n472 = event-data() -> ()  [unwired: 1 in, 5 out]
        n473 = call "函数类型1测试.vi"() -> ()  [unwired: 12 in]
      }
      event "btn_二维码识别": Value Change {
        n474 = event-data() -> ()  [unwired: 1 in, 5 out]
        n475 = call "生成板卡编号.vi"() -> ()  [unwired: 12 in]
      }
      event "函数类型 1": Mouse Leave {
        n476 = event-data() -> ()  [unwired: 1 in, 3 out]
        n477 = property on="函数类型 1" class="Bool"("Caption.Visible"=FALSE ("标签.可见")) -> ()  [unwired: 2 in, 2 out]
      }
      event "函数类型 1": Mouse Enter {
        n478 = event-data() -> ()  [unwired: 1 in, 3 out]
        n479 = property on="函数类型 1" class="Bool"("Caption.Visible"=TRUE ("标签.可见")) -> ()  [unwired: 2 in, 2 out]
      }
      event "函数类型 2": Value Change {
        n480 = event-data() -> ()  [unwired: 1 in, 5 out]
        n481 = call "函数类型2测试.vi"() -> ()  [unwired: 12 in]
      }
      event "函数类型 2": Mouse Enter {
        n482 = event-data() -> ()  [unwired: 1 in, 3 out]
        n483 = property on="函数类型 2" class="Bool"("Caption.Visible"=TRUE) -> ()  [unwired: 2 in, 2 out]
      }
      event "函数类型 2": Mouse Leave {
        n484 = event-data() -> ()  [unwired: 1 in, 3 out]
        n485 = property on="函数类型 2" class="Bool"("Caption.Visible"=FALSE) -> ()  [unwired: 2 in, 2 out]
      }
      event "函数类型 3": Value Change {
        n486 = event-data() -> ()  [unwired: 1 in, 5 out]
        n487 = call "函数类型3测试.vi"() -> ()  [unwired: 12 in]
      }
      event "函数类型 3": Mouse Enter {
        n488 = event-data() -> ()  [unwired: 1 in, 3 out]
        n489 = property on="函数类型 3" class="Bool"("Caption.Visible"=TRUE) -> ()  [unwired: 2 in, 2 out]
      }
      event "函数类型 3": Mouse Leave {
        n490 = event-data() -> ()  [unwired: 1 in, 3 out]
        n491 = property on="函数类型 3" class="Bool"("Caption.Visible"=FALSE) -> ()  [unwired: 2 in, 2 out]
      }
      event "函数类型 4": Value Change {
        n492 = event-data() -> ()  [unwired: 1 in, 5 out]
        n493 = call "函数类型4测试.vi"() -> ()  [unwired: 12 in]
      }
      event "函数类型 4": Mouse Enter {
        n494 = event-data() -> ()  [unwired: 1 in, 3 out]
        n495 = property on="函数类型 4" class="Bool"("Caption.Visible"=TRUE) -> ()  [unwired: 2 in, 2 out]
      }
      event "函数类型 4": Mouse Leave {
        n496 = event-data() -> ()  [unwired: 1 in, 3 out]
        n497 = property on="函数类型 4" class="Bool"("Caption.Visible"=FALSE) -> ()  [unwired: 2 in, 2 out]
      }
    }
    n498 = local write "退出？"(w143) -> ()
    n499 = Quit LabVIEW(quit? (T)=w143) -> ()
  }
  n500 = Obtain Notifier(name (unnamed)=w13, notification data type=w13) -> (notifier out=w12:refnum<notifier>, error out=w11:errorcluster)  [unwired: 2 in, 1 out]
  n501 = while {
    tunnel: w12 -> [w426]
    tunnel: w11 -> [w425]
    tunnel: [w424] -> w10
    tunnel: [w423] -> w9
    stop <- w418 stop-if-true
    # "I型板自动测试"
    n502 = Wait Until Next ms Multiple(millisecond multiple=u32 20 ("毫秒倍数")) -> ()  [unwired: 1 out]
    n503 = Wait on Notification(notifier=w426, timeout in ms (-1)=20 ("超时毫秒(-1)"), error in (no error)=w425) -> (notifier out=w424:refnum<notifier>, notification=w421:string, error out=w423:errorcluster)  [unwired: 1 in, 1 out]
    n504 = Equal?(x=w421, y="Auto" ("通知")) -> (x = y?=w420:bool)
    n505 = case shown="真" w420 {
      frame False {
      }
      frame True {
        n506 = stacked-sequence {
          frame #0 {
            # "数字量输入"
            n507 = local read "单选_数字量输入"() -> (w427:bool)
            n508 = stacked-sequence {
              tunnel: w427 -> [w429 w430]
              frame #0 {
                n509 = call "数字量输入自动检测.vi"("选择?"=w429) -> ()  [unwired: 11 in]
                n510 = local write "进度提示"("正在进行数字量输入测试......") -> ()
              }
              frame #1 {
                n511 = case shown="真" w430 {
                  frame False {
                  }
                  frame True {
                    n512 = global read "试验配置信息.vi" "自动检测结果"() -> (w432:bool[])
                    n513 = Index Array(array=w432, index=0) -> (element=w434:bool)
                    n514 = case shown="真" w434 {
                      tunnel: [2 1] -> w435
                      frame False {
                      }
                      frame True {
                      }
                    }
                    n515 = case shown="0, 默认" w435 {
                      tunnel: [cluster{u32, u32}[] [{1985280, 1985280}] cluster{u32, u32}[] [{61205, 6618880}] cluster{u32, u32}[] [{16730410, 16711680}]] -> w431
                      frame 0, Default {
                      }
                      frame 1 {
                      }
                      frame 2 {
                      }
                    }
                    n516 = property on="数字量输入检测" class="Bool (严格)"("Colors [4]"=w431) -> ()  [unwired: 2 in, 2 out]
                  }
                }
              }
            }
          }
          frame #1 {
            # "数字量输出"
            n517 = local read "单选_数字量输出"() -> (w441:bool)
            n518 = stacked-sequence {
              tunnel: w441 -> [w443 w444]
              frame #0 {
                n519 = call "自动数量输出.vi"("选择？"=w443) -> ()  [unwired: 11 in]
                n520 = local write "进度提示"("正在进行数字量输出测试......") -> ()
              }
              frame #1 {
                n521 = case shown="真" w444 {
                  frame False {
                  }
                  frame True {
                    n522 = global read "试验配置信息.vi" "自动检测结果"() -> (w446:bool[])
                    n523 = Index Array(array=w446, index=1) -> (element=w448:bool)
                    n524 = case shown="假" w448 {
                      tunnel: [2 1] -> w449
                      frame False {
                      }
                      frame True {
                      }
                    }
                    n525 = case shown="0, 默认" w449 {
                      tunnel: [cluster{u32, u32}[] [{1985280, 1985280}] cluster{u32, u32}[] [{61205, 6618880}] cluster{u32, u32}[] [{16730410, 16711680}]] -> w445
                      frame 0, Default {
                      }
                      frame 1 {
                      }
                      frame 2 {
                      }
                    }
                    n526 = property on="数字量输出检测" class="Bool (严格)"("Colors [4]"=w445) -> ()  [unwired: 2 in, 2 out]
                  }
                }
              }
            }
          }
          frame #2 {
            # "模拟量输入"
            n527 = local read "单选_DSP输入"() -> (w456:bool)
            n528 = property on="单选_AD输入" class="Bool (严格)"() -> ("Value"=w455:bool)  [unwired: 2 in, 2 out]
            n529 = stacked-sequence {
              tunnel: w456 -> [w459 w461]
              tunnel: w455 -> [w458 w460]
              frame #0 {
                n530 = call "模拟量输入自动测试.vi"("AD选择?"=w458, "DSP选择?"=w459) -> ()  [unwired: 10 in]
                n531 = local write "进度提示"("正在进行模拟量测试......") -> ()
              }
              frame #1 {
                n532 = stacked-sequence {
                  tunnel: w461 -> [w462 _]
                  tunnel: w460 -> [_ w473]
                  frame #0 {
                    n533 = case shown="真" w462 {
                      frame False {
                      }
                      frame True {
                        n534 = global read "试验配置信息.vi" "自动检测结果"() -> (w464:bool[])
                        n535 = Index Array(array=w464, index=2) -> (element=w466:bool)
                        n536 = case shown="假" w466 {
                          tunnel: [2 1] -> w467
                          frame False {
                          }
                          frame True {
                          }
                        }
                        n537 = case shown="0, 默认" w467 {
                          tunnel: [cluster{u32, u32}[] [{1985280, 1985280}] cluster{u32, u32}[] [{61205, 6618880}] cluster{u32, u32}[] [{16730410, 16711680}]] -> w463
                          frame 0, Default {
                          }
                          frame 1 {
                          }
                          frame 2 {
                          }
                        }
                        n538 = property on="模拟量DSP输入检测" class="Bool (严格)"("Colors [4]"=w463) -> ()  [unwired: 2 in, 2 out]
                      }
                    }
                  }
                  frame #1 {
                    n539 = case shown="真" w473 {
                      frame False {
                      }
                      frame True {
                        n540 = global read "试验配置信息.vi" "自动检测结果"() -> (w475:bool[])
                        n541 = Index Array(array=w475, index=3) -> (element=w477:bool)
                        n542 = case shown="假" w477 {
                          tunnel: [2 1] -> w478
                          frame False {
                          }
                          frame True {
                          }
                        }
                        n543 = case shown="0, 默认" w478 {
                          tunnel: [cluster{u32, u32}[] [{1985280, 1985280}] cluster{u32, u32}[] [{61205, 6618880}] cluster{u32, u32}[] [{16730410, 16711680}]] -> w474
                          frame 0, Default {
                          }
                          frame 1 {
                          }
                          frame 2 {
                          }
                        }
                        n544 = property on="模拟量AD输入检测" class="Bool (严格)"("Colors [4]"=w474) -> ()  [unwired: 2 in, 2 out]
                      }
                    }
                  }
                }
              }
            }
          }
          frame #3 {
            # "串口"
            n545 = local read "单选_R232检测"() -> (w485:bool)
            n546 = local read "单选_R485检测"() -> (w484:bool)
            n547 = stacked-sequence {
              tunnel: w485 -> [w488 w490]
              tunnel: w484 -> [w487 w489]
              frame #0 {
                n548 = call "串口自动测试.vi"("RS485选择"=w487, "RS232选择"=w488) -> ()  [unwired: 10 in]
                n549 = local write "进度提示"("正在进行串口测试......") -> ()
              }
              frame #1 {
                n550 = stacked-sequence {
                  tunnel: w490 -> [w491 _]
                  tunnel: w489 -> [_ w502]
                  frame #0 {
                    n551 = case shown="真" w491 {
                      frame False {
                      }
                      frame True {
                        n552 = global read "试验配置信息.vi" "自动检测结果"() -> (w493:bool[])
                        n553 = Index Array(array=w493, index=4) -> (element=w495:bool)
                        n554 = case shown="假" w495 {
                          tunnel: [2 1] -> w496
                          frame False {
                          }
                          frame True {
                          }
                        }
                        n555 = case shown="0, 默认" w496 {
                          tunnel: [cluster{u32, u32}[] [{1985280, 1985280}] cluster{u32, u32}[] [{61205, 6618880}] cluster{u32, u32}[] [{16730410, 16711680}]] -> w492
                          frame 0, Default {
                          }
                          frame 1 {
                          }
                          frame 2 {
                          }
                        }
                        n556 = property on="RS232总线检测" class="Bool (严格)"("Colors [4]"=w492) -> ()  [unwired: 2 in, 2 out]
                      }
                    }
                  }
                  frame #1 {
                    n557 = case shown="真" w502 {
                      frame False {
                      }
                      frame True {
                        n558 = global read "试验配置信息.vi" "自动检测结果"() -> (w504:bool[])
                        n559 = Index Array(array=w504, index=5) -> (element=w506:bool)
                        n560 = case shown="假" w506 {
                          tunnel: [2 1] -> w507
                          frame False {
                          }
                          frame True {
                          }
                        }
                        n561 = case shown="0, 默认" w507 {
                          tunnel: [cluster{u32, u32}[] [{1985280, 1985280}] cluster{u32, u32}[] [{61205, 6618880}] cluster{u32, u32}[] [{16730410, 16711680}]] -> w503
                          frame 0, Default {
                          }
                          frame 1 {
                          }
                          frame 2 {
                          }
                        }
                        n562 = property on="RS485总线检测" class="Bool (严格)"("Colors [4]"=w503) -> ()  [unwired: 2 in, 2 out]
                      }
                    }
                  }
                }
              }
            }
          }
          frame #4 {
            # "CAN"
            n563 = local read "单选_CAN检测"() -> (w513:bool)
            n564 = stacked-sequence {
              tunnel: w513 -> [w515 w516]
              frame #0 {
                n565 = call "CAN自动测试.vi"("选择?"=w515) -> ()  [unwired: 11 in]
                n566 = local write "进度提示"("正在进行CAN测试......") -> ()
              }
              frame #1 {
                n567 = case shown="真" w516 {
                  frame False {
                  }
                  frame True {
                    n568 = global read "试验配置信息.vi" "自动检测结果"() -> (w518:bool[])
                    n569 = Index Array(array=w518, index=6) -> (element=w520:bool)
                    n570 = case shown="假" w520 {
                      tunnel: [2 1] -> w521
                      frame False {
                      }
                      frame True {
                      }
                    }
                    n571 = case shown="0, 默认" w521 {
                      tunnel: [cluster{u32, u32}[] [{1985280, 1985280}] cluster{u32, u32}[] [{61205, 6618880}] cluster{u32, u32}[] [{16730410, 16711680}]] -> w517
                      frame 0, Default {
                      }
                      frame 1 {
                      }
                      frame 2 {
                      }
                    }
                    n572 = property on="CAN总线检测" class="Bool (严格)"("Colors [4]"=w517) -> ()  [unwired: 2 in, 2 out]
                  }
                }
              }
            }
          }
          frame #5 {
            # "以太网"
            n573 = local read "单选_LAN检测"() -> (w527:bool)
            n574 = stacked-sequence {
              tunnel: w527 -> [w529 w530]
              frame #0 {
                n575 = call "以太网自动测试.vi"("选择?"=w529) -> ()  [unwired: 11 in]
                n576 = local write "进度提示"("正在进行LAN测试......") -> ()
              }
              frame #1 {
                n577 = case shown="真" w530 {
                  frame False {
                  }
                  frame True {
                    n578 = global read "试验配置信息.vi" "自动检测结果"() -> (w532:bool[])
                    n579 = Index Array(array=w532, index=7) -> (element=w534:bool)
                    n580 = case shown="假" w534 {
                      tunnel: [2 1] -> w535
                      frame False {
                      }
                      frame True {
                      }
                    }
                    n581 = case shown="0, 默认" w535 {
                      tunnel: [cluster{u32, u32}[] [{1985280, 1985280}] cluster{u32, u32}[] [{61205, 6618880}] cluster{u32, u32}[] [{16730410, 16711680}]] -> w531
                      frame 0, Default {
                      }
                      frame 1 {
                      }
                      frame 2 {
                      }
                    }
                    n582 = property on="LAN总线检测" class="Bool (严格)"("Colors [4]"=w531) -> ()  [unwired: 2 in, 2 out]
                  }
                }
              }
            }
          }
          frame #6 {
            # "统计合格率"
            n583 = call "统计合格率.vi"() -> ()  [unwired: 12 in]
          }
          frame #7 {
            n584 = flat-sequence {
              frame #0 {
                # "报告存储"
                n585 = Get Date/Time In Seconds() -> (seconds since 1Jan1904=w541:timestamp)
                n586 = call "报告存储.vi"("试验时间"=w541) -> ()  [unwired: 11 in]
              }
              frame #1 {
                n587 = call "完成"() -> ()  [unwired: 10 in, 2 out]
              }
            }
            n588 = disable-structure shown="禁用" {
              frame Disabled {
                n589 = Get Date/Time In Seconds() -> (seconds since 1Jan1904=w542:timestamp)
                n590 = call "测试报告摘要4.vi"("打印?"=FALSE, "试验时间"=w542) -> ()  [unwired: 10 in]
              }
              frame Enabled {
              }
            }
          }
          frame #8 {
            w545 = T3."Enabled" ("禁用")
            n591 = case shown="0, 默认" 0 {
              tunnel: [cluster{u32, u32}[] [{1985280, 1985280}] cluster{u32, u32}[] [{61205, 6618880}] cluster{u32, u32}[] [{16730410, 16711680}]] -> w546
              frame 0, Default {
              }
              frame 1 {
              }
              frame 2 {
              }
            }
            n592 = property on="数字量输入检测" class="Bool (严格)"("Colors [4]"=w546) -> ()  [unwired: 2 in, 2 out]
            n593 = property on="数字量输出检测" class="Bool (严格)"("Colors [4]"=w546) -> ()  [unwired: 2 in, 2 out]
            n594 = property on="模拟量AD输入检测" class="Bool (严格)"("Colors [4]"=w546) -> ()  [unwired: 2 in, 2 out]
            n595 = property on="CAN总线检测" class="Bool (严格)"("Colors [4]"=w546) -> ()  [unwired: 2 in, 2 out]
            n596 = local write "进度提示"("测试完毕......") -> ()
            n597 = property on="LAN总线检测" class="Bool (严格)"("Colors [4]"=w546) -> ()  [unwired: 2 in, 2 out]
            n598 = property on="RS232总线检测" class="Bool (严格)"("Colors [4]"=w546) -> ()  [unwired: 2 in, 2 out]
            n599 = property on="RS485总线检测" class="Bool (严格)"("Colors [4]"=w546) -> ()  [unwired: 2 in, 2 out]
            n600 = property on="模拟量DSP输入检测" class="Bool (严格)"("Colors [4]"=w546) -> ()  [unwired: 2 in, 2 out]
            n601 = property on="btn_数字输入" class="Bool"("DisabledEnum"=w545) -> ()  [unwired: 2 in, 2 out]
            n602 = property on="btn_数字输出" class="Bool"("DisabledEnum"=w545) -> ()  [unwired: 2 in, 2 out]
            n603 = property on="btn_DSP输入" class="Bool"("DisabledEnum"=w545) -> ()  [unwired: 2 in, 2 out]
            n604 = property on="btn_CAN总线" class="Bool"("DisabledEnum"=w545) -> ()  [unwired: 2 in, 2 out]
            n605 = property on="btn_R232_485总线" class="Bool"("DisabledEnum"=w545) -> ()  [unwired: 2 in, 2 out]
            n606 = property on="btn_LAN总线" class="Bool"("DisabledEnum"=w545) -> ()  [unwired: 2 in, 2 out]
            n607 = property on="btn_自动开始检测类型2" class="Bool"("DisabledEnum"=w545) -> ()  [unwired: 2 in, 2 out]
            n608 = property on="函数类型 1" class="Bool"("DisabledEnum"=w545) -> ()  [unwired: 2 in, 2 out]
            n609 = property on="函数类型 2" class="Bool"("DisabledEnum"=w545) -> ()  [unwired: 2 in, 2 out]
            n610 = property on="函数类型 3" class="Bool"("DisabledEnum"=w545) -> ()  [unwired: 2 in, 2 out]
            n611 = property on="函数类型 4" class="Bool"("DisabledEnum"=w545) -> ()  [unwired: 2 in, 2 out]
          }
        }
      }
    }
    n612 = local read "退出？"() -> (w418:bool)
  }
  n613 = Obtain Notifier(name (unnamed)=w8, notification data type=w8) -> (notifier out=w7:refnum<notifier>, error out=w6:errorcluster)  [unwired: 2 in, 1 out]
  n614 = while {
    tunnel: w7 -> [w560]
    tunnel: w6 -> [w559]
    tunnel: [w558] -> w5
    tunnel: [w557] -> w4
    stop <- w551 stop-if-true
    # "II型板自动测试"
    n615 = Wait Until Next ms Multiple(millisecond multiple=u32 20 ("毫秒倍数")) -> ()  [unwired: 1 out]
    n616 = Wait on Notification(notifier=w560, timeout in ms (-1)=20 ("超时毫秒(-1)"), error in (no error)=w559) -> (notifier out=w558:refnum<notifier>, notification=w555:string, error out=w557:errorcluster)  [unwired: 1 in, 1 out]
    n617 = Equal?(x=w555, y="Auto_2" ("通知")) -> (x = y?=w552:bool)
    n618 = case shown="真" w552 {
      frame False {
      }
      frame True {
        n619 = stacked-sequence {
          frame #0 {
            # "类型1测试"
            n620 = local read "单选_函数类型1"() -> (w561:bool)
            n621 = case shown="真" w561 {
              frame False {
              }
              frame True {
                n622 = stacked-sequence {
                  frame #0 {
                    n623 = stacked-sequence {
                      frame #0 {
                        n624 = call "测试类型1自动测试一组.vi"() -> ()  [unwired: 10 in]
                      }
                      frame #1 {
                        n625 = call "自动测试类型1统计结果.vi"() -> ()  [unwired: 12 in]
                      }
                    }
                    n626 = local write "进度提示"("正在进行类型1测试......") -> ()
                  }
                  frame #1 {
                    n627 = global read "试验配置信息.vi" "板卡II自动检测结果"() -> (w566:bool[])
                    n628 = Index Array(array=w566, index=0) -> (element=w564:bool)
                    n629 = case shown="假" w564 {
                      tunnel: [2 1] -> w563
                      frame False {
                      }
                      frame True {
                      }
                    }
                    n630 = case shown="0, 默认" w563 {
                      tunnel: [cluster{u32, u32}[] [{1985280, 1985280}] cluster{u32, u32}[] [{61205, 6618880}] cluster{u32, u32}[] [{16730410, 16711680}]] -> w567
                      frame 0, Default {
                      }
                      frame 1 {
                      }
                      frame 2 {
                      }
                    }
                    n631 = property on="函数类型1检测" class="Bool (严格)"("Colors [4]"=w567) -> ()  [unwired: 2 in, 2 out]
                  }
                }
              }
            }
          }
          frame #1 {
            # "类型2测试"
            n632 = stacked-sequence {
              frame #0 {
                n633 = stacked-sequence {
                  frame #0 {
                    n634 = call "类型2自动测试.vi"() -> ()  [unwired: 12 in]
                  }
                  frame #1 {
                    n635 = call "自动测试类型2统计结果.vi"() -> ()  [unwired: 12 in]
                  }
                }
                n636 = local write "进度提示"("正在进行类型2测试......") -> ()
              }
              frame #1 {
                n637 = global read "试验配置信息.vi" "板卡II自动检测结果"() -> (w577:bool[])
                n638 = Index Array(array=w577, index=1) -> (element=w575:bool)
                n639 = case shown="假" w575 {
                  tunnel: [2 1] -> w574
                  frame False {
                  }
                  frame True {
                  }
                }
                n640 = case shown="0, 默认" w574 {
                  tunnel: [cluster{u32, u32}[] [{1985280, 1985280}] cluster{u32, u32}[] [{61205, 6618880}] cluster{u32, u32}[] [{16730410, 16711680}]] -> w578
                  frame 0, Default {
                  }
                  frame 1 {
                  }
                  frame 2 {
                  }
                }
                n641 = property on="函数类型2检测" class="Bool (严格)"("Colors [4]"=w578) -> ()  [unwired: 2 in, 2 out]
              }
            }
          }
          frame #2 {
            # "类型3测试"
            n642 = local read "单选_函数类型3"() -> (w584:bool)
            n643 = stacked-sequence {
              tunnel: w584 -> [w586 _]
              frame #0 {
                n644 = call "类型3自动测试.vi"("选择?"=w586) -> ()  [unwired: 11 in]
                n645 = local write "进度提示"("正在进行类型3测试......") -> ()
              }
              frame #1 {
                n646 = global read "试验配置信息.vi" "板卡II自动检测结果"() -> (w590:bool[])
                n647 = Index Array(array=w590, index=2) -> (element=w588:bool)
                n648 = case shown="假" w588 {
                  tunnel: [2 1] -> w587
                  frame False {
                  }
                  frame True {
                  }
                }
                n649 = case shown="0, 默认" w587 {
                  tunnel: [cluster{u32, u32}[] [{1985280, 1985280}] cluster{u32, u32}[] [{61205, 6618880}] cluster{u32, u32}[] [{16730410, 16711680}]] -> w591
                  frame 0, Default {
                  }
                  frame 1 {
                  }
                  frame 2 {
                  }
                }
                n650 = property on="函数类型3检测" class="Bool (严格)"("Colors [4]"=w591) -> ()  [unwired: 2 in, 2 out]
              }
            }
          }
          frame #3 {
            # "类型4测试"
            n651 = stacked-sequence {
              frame #0 {
                n652 = local write "进度提示"("正在进行类型4测试......") -> ()
              }
              frame #1 {
                n653 = global read "试验配置信息.vi" "板卡II自动检测结果"() -> (w601:bool[])
                n654 = Index Array(array=w601, index=3) -> (element=w599:bool)
                n655 = case shown="假" w599 {
                  tunnel: [2 1] -> w598
                  frame False {
                  }
                  frame True {
                  }
                }
                n656 = case shown="0, 默认" w598 {
                  tunnel: [cluster{u32, u32}[] [{1985280, 1985280}] cluster{u32, u32}[] [{61205, 6618880}] cluster{u32, u32}[] [{16730410, 16711680}]] -> w602
                  frame 0, Default {
                  }
                  frame 1 {
                  }
                  frame 2 {
                  }
                }
                n657 = property on="函数类型4检测" class="Bool (严格)"("Colors [4]"=w602) -> ()  [unwired: 2 in, 2 out]
              }
            }
          }
          frame #4 {
            # "统计合格率"
            n658 = call "二型板自动测试合格率统计.vi"() -> ()  [unwired: 12 in]
          }
          frame #5 {
            # "报告存储"
            n659 = flat-sequence {
              frame #0 {
                n660 = Get Date/Time In Seconds() -> (seconds since 1Jan1904=w608:timestamp)
                n661 = call "二型板测试报告存储.vi"("试验时间"=w608) -> ()  [unwired: 11 in]
              }
              frame #1 {
                n662 = call "完成2"() -> ()  [unwired: 10 in, 2 out]
              }
            }
          }
          frame #6 {
            w610 = T3."Enabled" ("禁用")
            n663 = case shown="0, 默认" 0 {
              tunnel: [cluster{u32, u32}[] [{1985280, 1985280}] cluster{u32, u32}[] [{61205, 6618880}] cluster{u32, u32}[] [{16730410, 16711680}]] -> w612
              frame 0, Default {
              }
              frame 1 {
              }
              frame 2 {
              }
            }
            n664 = property on="函数类型1检测" class="Bool (严格)"("Colors [4]"=w612) -> ()  [unwired: 2 in, 2 out]
            n665 = property on="函数类型2检测" class="Bool (严格)"("Colors [4]"=w612) -> ()  [unwired: 2 in, 2 out]
            n666 = property on="函数类型3检测" class="Bool (严格)"("Colors [4]"=w612) -> ()  [unwired: 2 in, 2 out]
            n667 = property on="函数类型4检测" class="Bool (严格)"("Colors [4]"=w612) -> ()  [unwired: 2 in, 2 out]
            n668 = local write "进度提示"("测试完毕......") -> ()
            n669 = property on="btn_数字输入" class="Bool"("DisabledEnum"=w610) -> ()  [unwired: 2 in, 2 out]
            n670 = property on="btn_数字输出" class="Bool"("DisabledEnum"=w610) -> ()  [unwired: 2 in, 2 out]
            n671 = property on="btn_DSP输入" class="Bool"("DisabledEnum"=w610) -> ()  [unwired: 2 in, 2 out]
            n672 = property on="btn_CAN总线" class="Bool"("DisabledEnum"=w610) -> ()  [unwired: 2 in, 2 out]
            n673 = property on="btn_R232_485总线" class="Bool"("DisabledEnum"=w610) -> ()  [unwired: 2 in, 2 out]
            n674 = property on="btn_LAN总线" class="Bool"("DisabledEnum"=w610) -> ()  [unwired: 2 in, 2 out]
            n675 = property on="函数类型 1" class="Bool"("DisabledEnum"=w610) -> ()  [unwired: 2 in, 2 out]
            n676 = property on="函数类型 2" class="Bool"("DisabledEnum"=w610) -> ()  [unwired: 2 in, 2 out]
            n677 = property on="函数类型 3" class="Bool"("DisabledEnum"=w610) -> ()  [unwired: 2 in, 2 out]
            n678 = property on="函数类型 4" class="Bool"("DisabledEnum"=w610) -> ()  [unwired: 2 in, 2 out]
            n679 = property on="btn_开始检测" class="Bool"("DisabledEnum"=w610) -> ()  [unwired: 2 in, 2 out]
          }
        }
      }
    }
    n680 = local read "退出？"() -> (w551:bool)
  }
  n681 = Release Notifier(notifier=w10, error in (no error)=w9) -> ()  [unwired: 1 in, 3 out]
  n682 = Release Notifier(notifier=w5, error in (no error)=w4) -> ()  [unwired: 1 in, 3 out]
